vi "CAN CONF.vi"() -> ()   [LabVIEW 2018]
uses:
  Controls/CLUSTER.ctl
  Controls/FEV_DBC CLUSTER.ctl
  Controls/DBC CLUSTER.ctl
  <resource>/objmgr/xnet.rc
panel:
  out "File paths.Model File path":path
  out "appended path":path
  in  "DBC FUNCTIONS":T1[](array[typedef])
  out "Headline":string
  in  "ADD":bool
  in  "Save Button":bool
  in  "ALL DBC FUNCTIONS":T3[](array[typedef])
  in  "DBC File Selection":refnum<k21>="CAN DATA"
  out "Frames":refnum<k21>[](array[refnum])
  in  "MODEL SELECTION":string(combo)
  # "FUNCTIONS"
  # "FUNCTIONS"
  # "READ"
  # "WRITE"
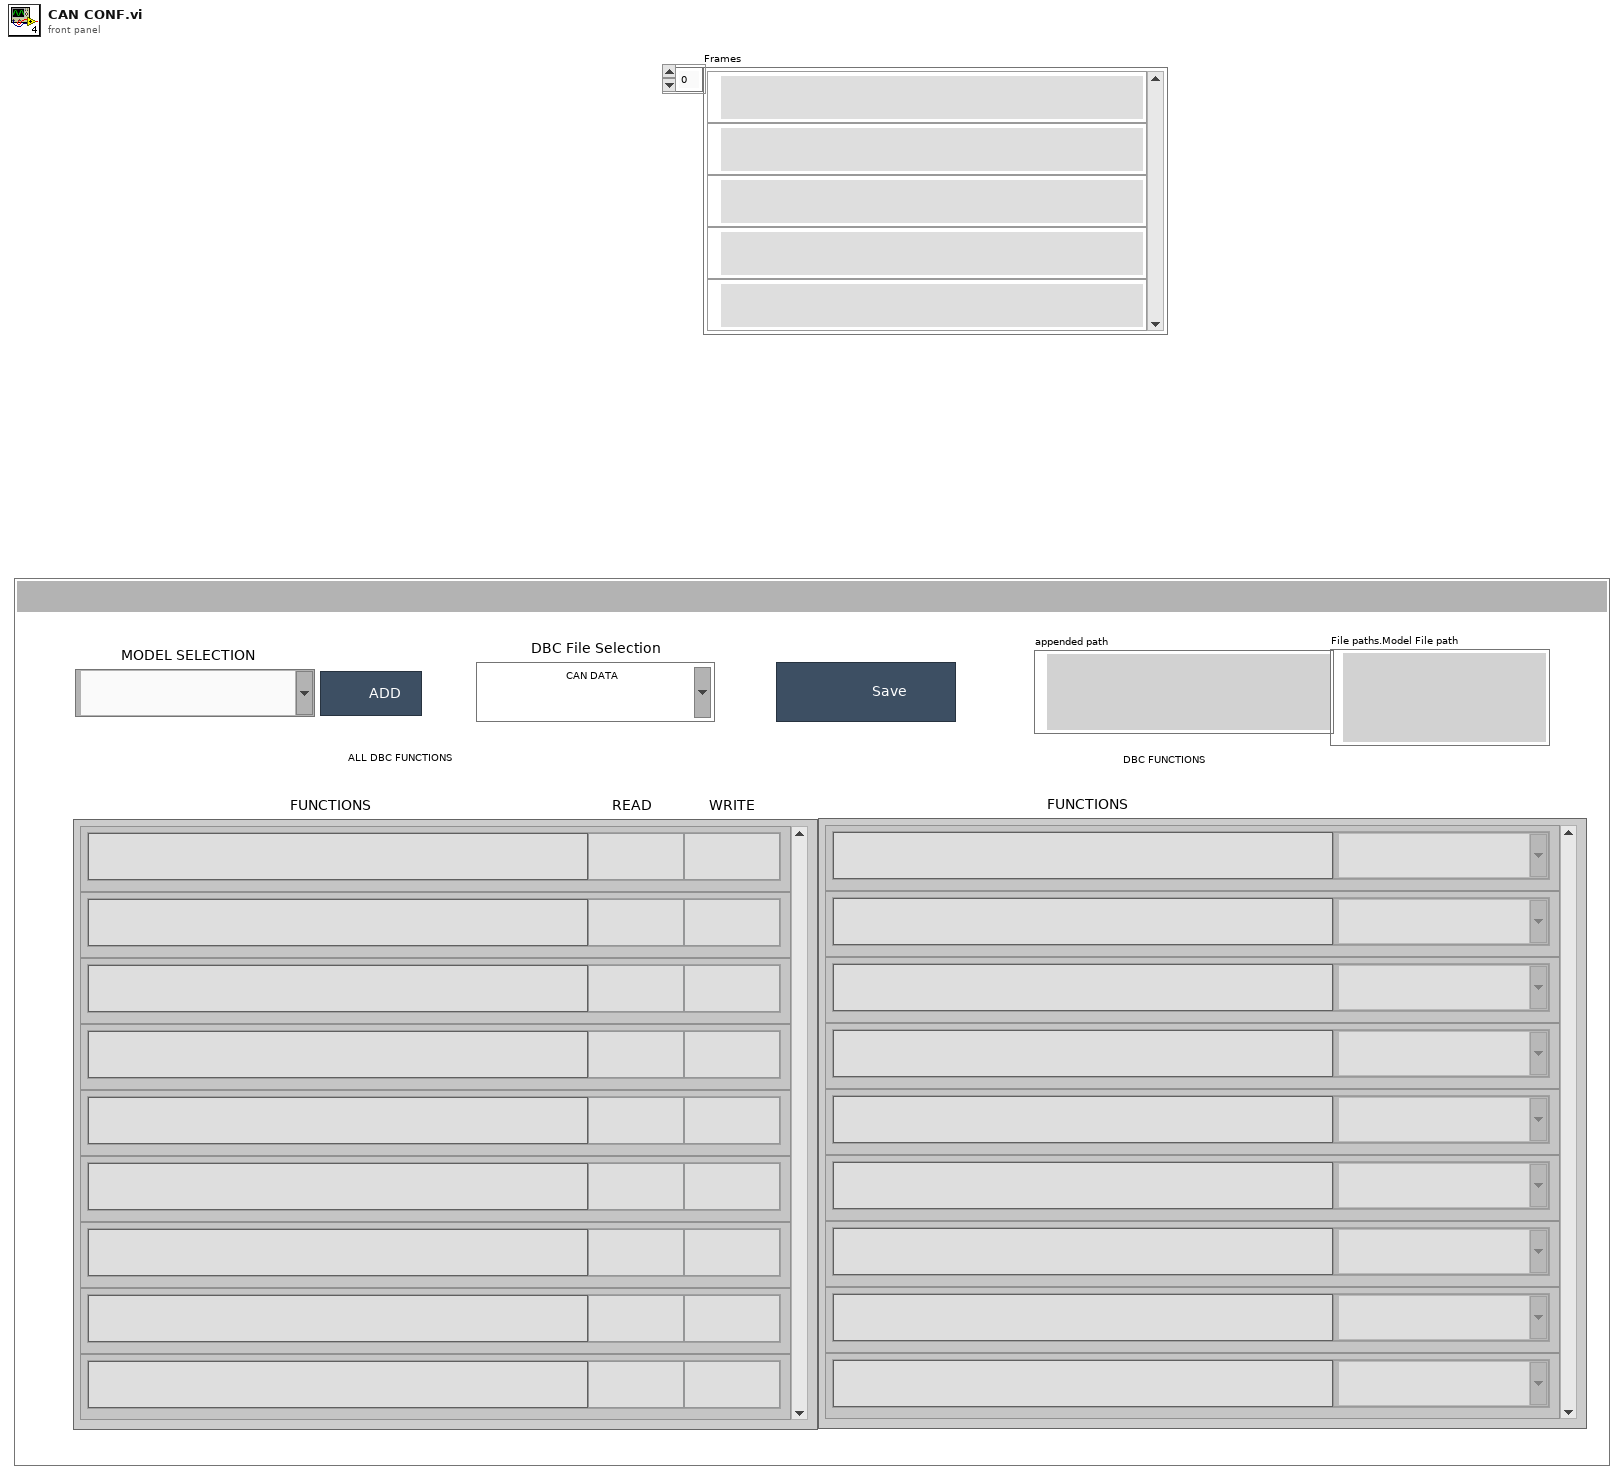
[diagram p1: front panel]
types:
  T1 = typedef "FEV_DBC CLUSTER.ctl" = cluster{"FUNCTION":T2, "DYNO FUNCTION":string}
  T2 = typedef "DBC CLUSTER.ctl" = string
  T3 = typedef "CLUSTER.ctl" = cluster{"FUNCTION":string, "READ":bool, "WRITE":bool}
  T4 = enum32{"Invalid", "Standard", "Closed", "Hidden", "Minimized", "Maximized"}
  T5 = enum32{"invalid app kind", "Development System", "Run Time System", "Student Edition", "Embedded LabVIEW", "Evaluation", "Custom"}
  T6 = cluster{"Core":cluster{"Current VI Reference":refnum<vi>, "Close Panel on Exit?":bool}, "Your Boolean data":bool, "Your string data":string, "ALL DBC FUNCTIONS":T3[], "File paths":cluster{"Base file path":path, "Model File path":path}, "DBC FUNCTIONS":T1[]}
  T7 = cluster{"Base file path":path, "Model File path":path}
  T8 = cluster{"Current VI Reference":refnum<vi>, "Close Panel on Exit?":bool}
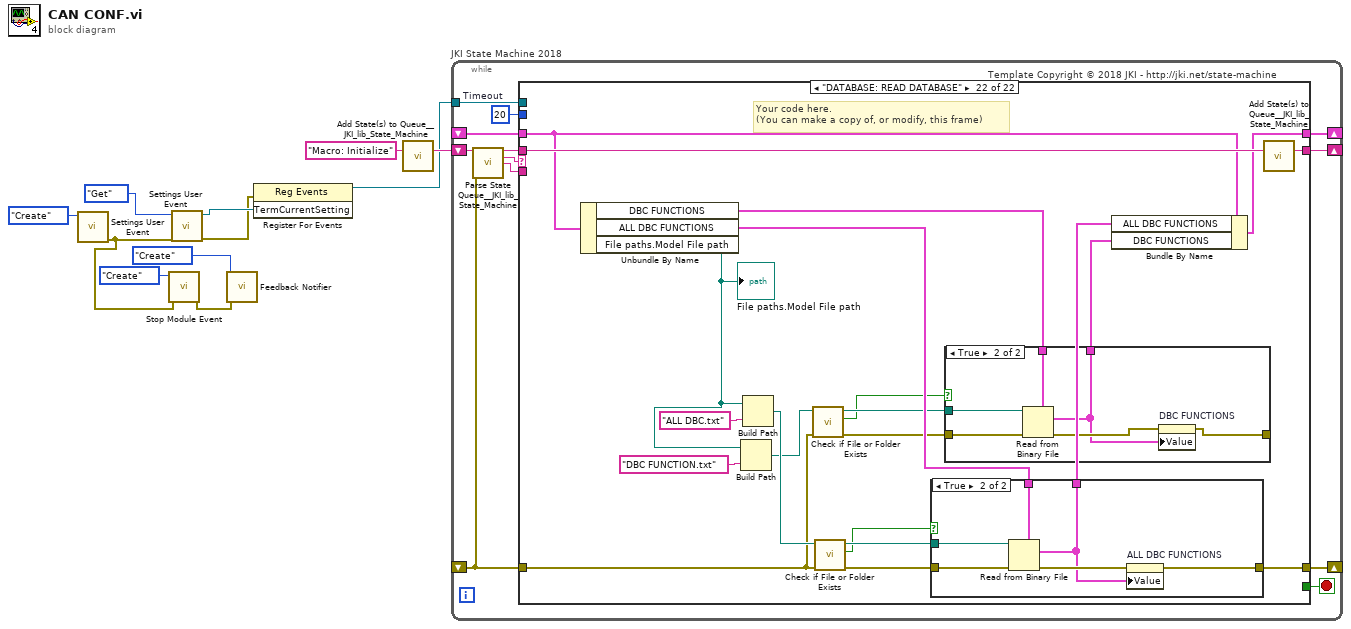
[diagram p0: block diagram]
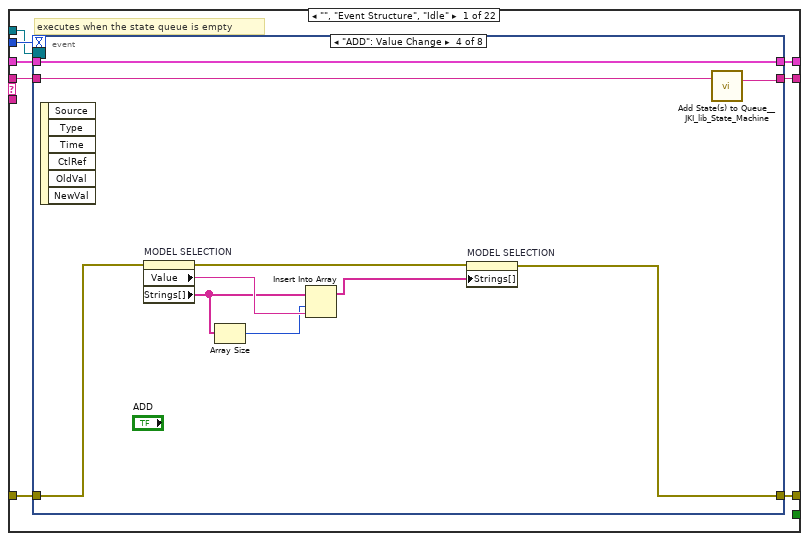
[diagram p2: hidden frame]
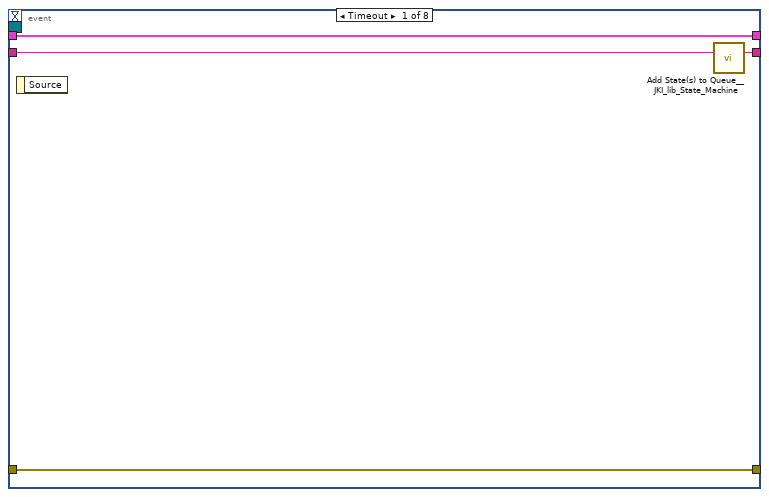
[diagram p3: hidden frame]
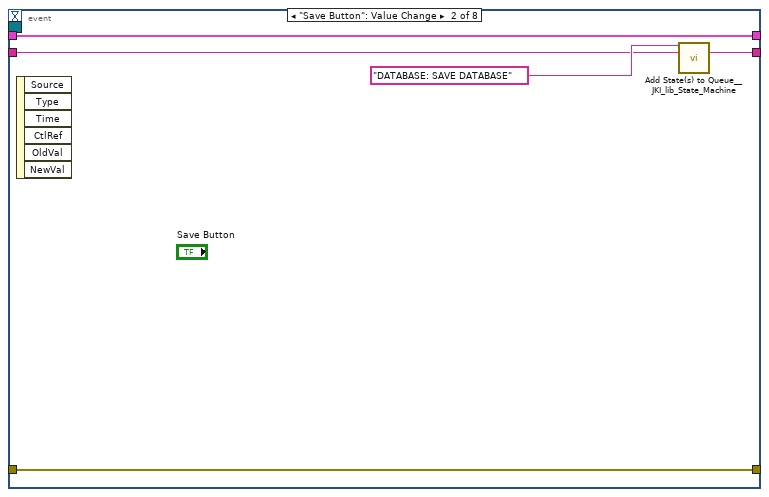
[diagram p4: hidden frame]
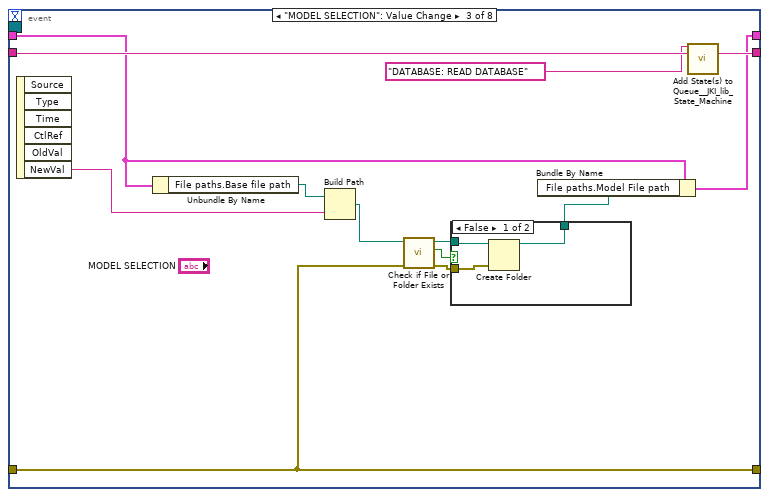
[diagram p5: hidden frame]
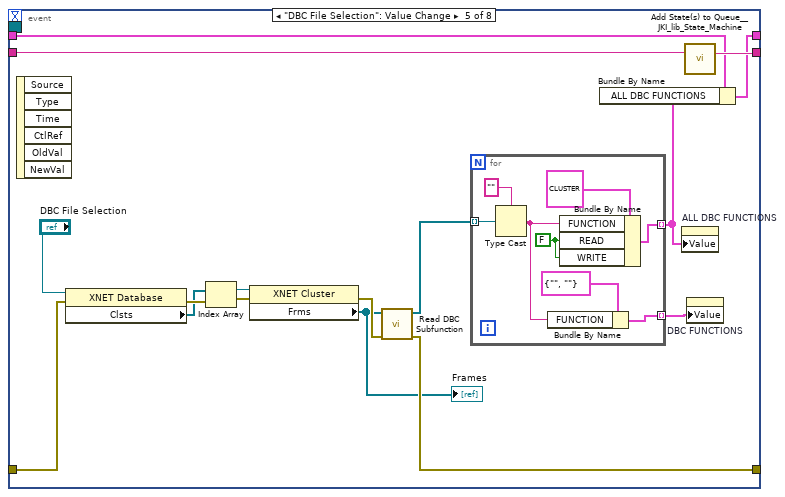
[diagram p7: hidden frame]
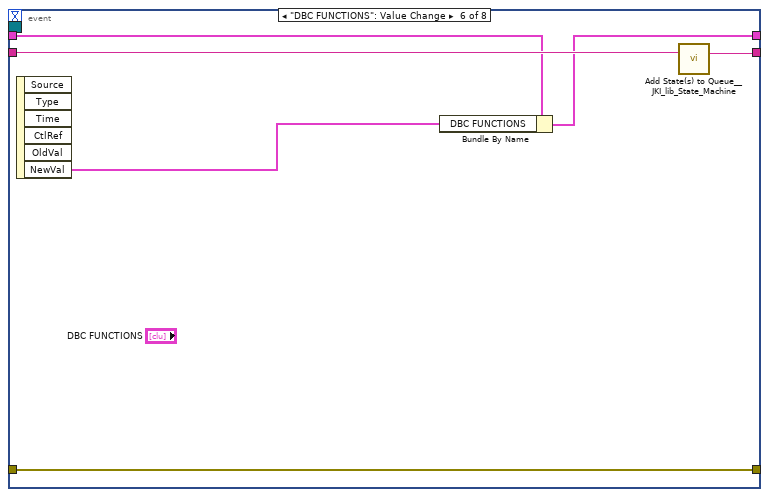
[diagram p8: hidden frame]
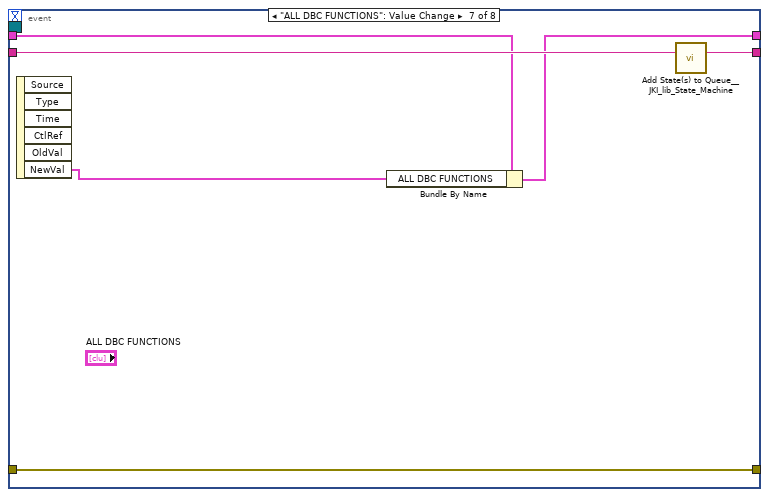
[diagram p9: hidden frame]
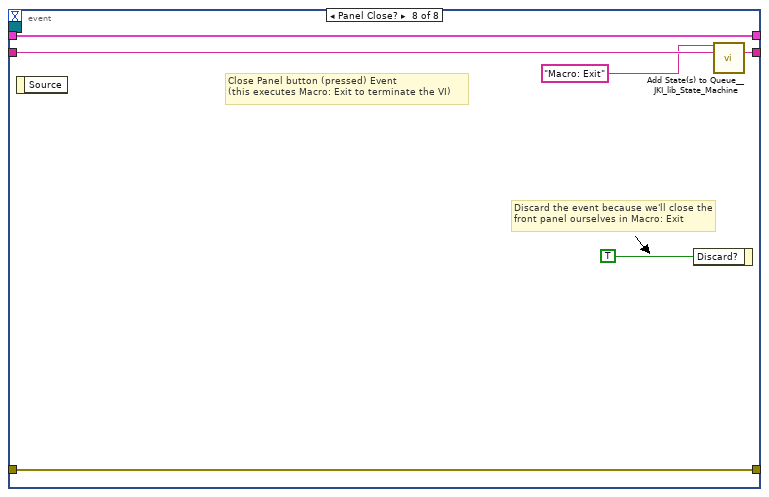
[diagram p10: hidden frame]
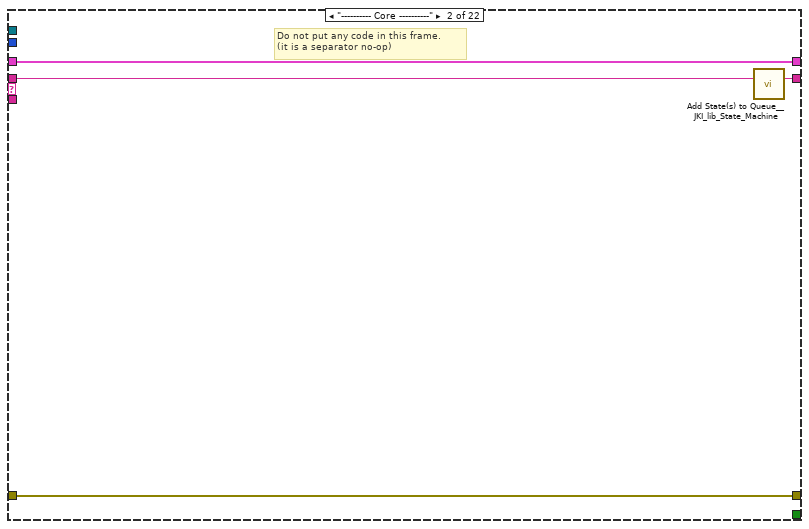
[diagram p11: hidden frame]
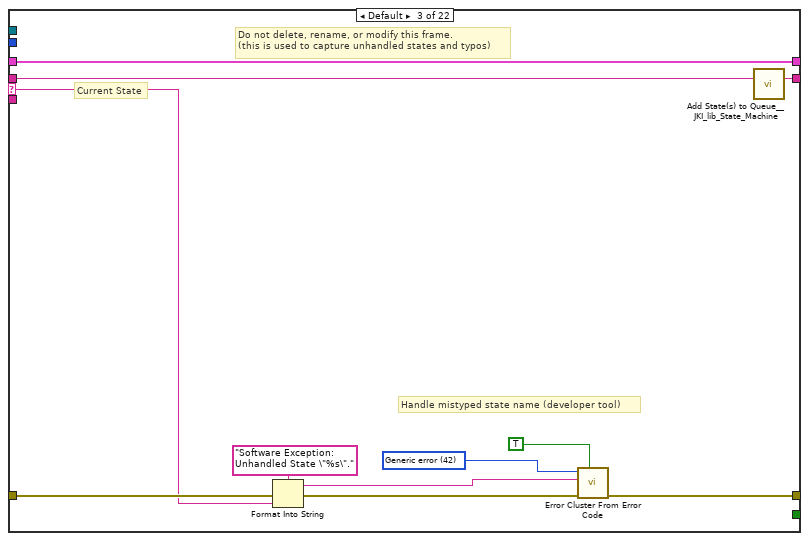
[diagram p12: hidden frame]
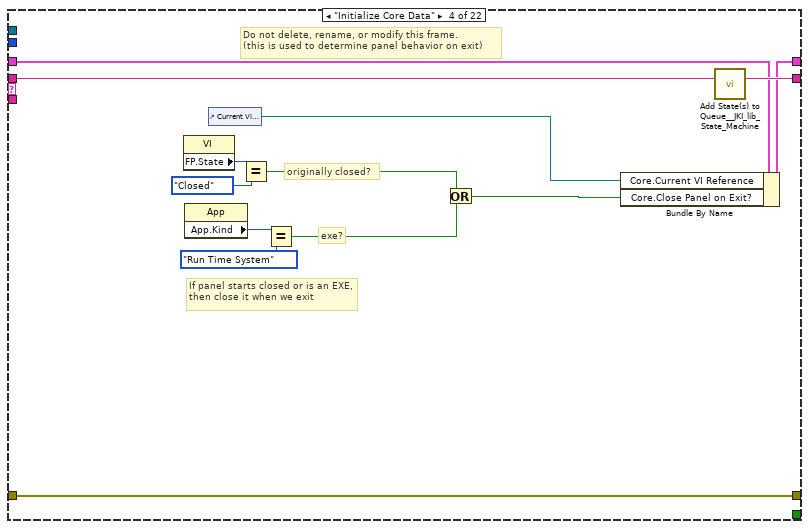
[diagram p13: hidden frame]
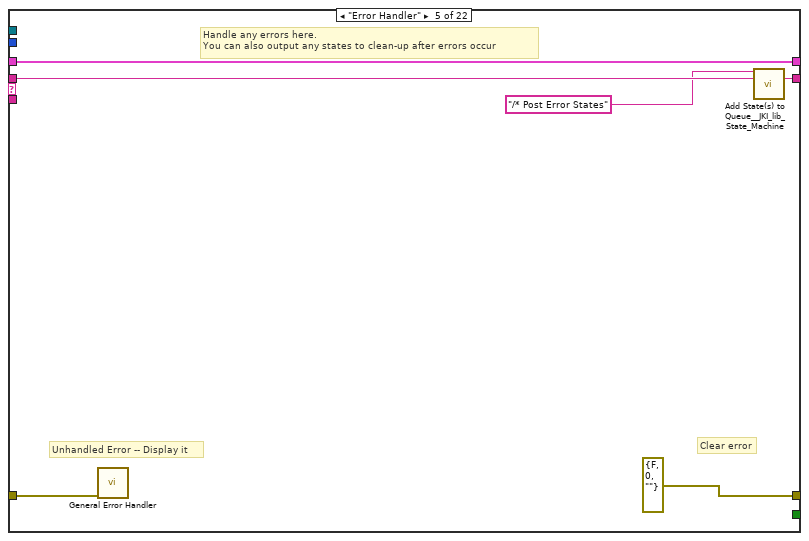
[diagram p14: hidden frame]
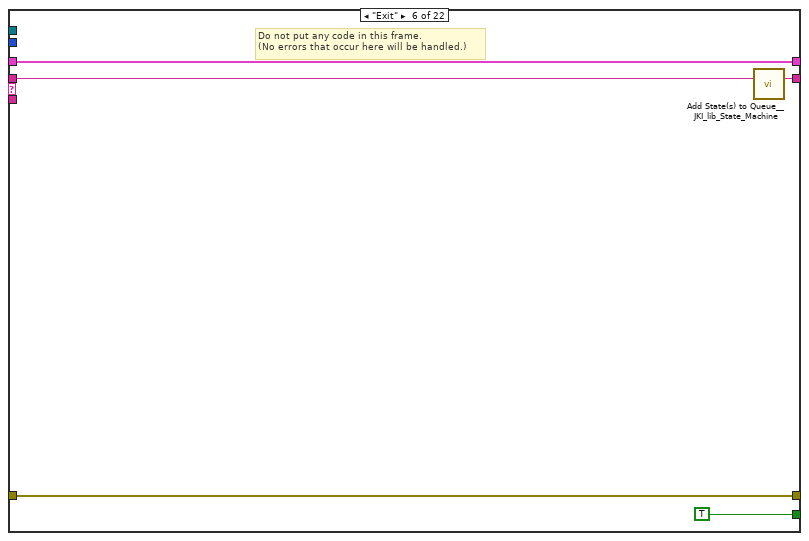
[diagram p15: hidden frame]
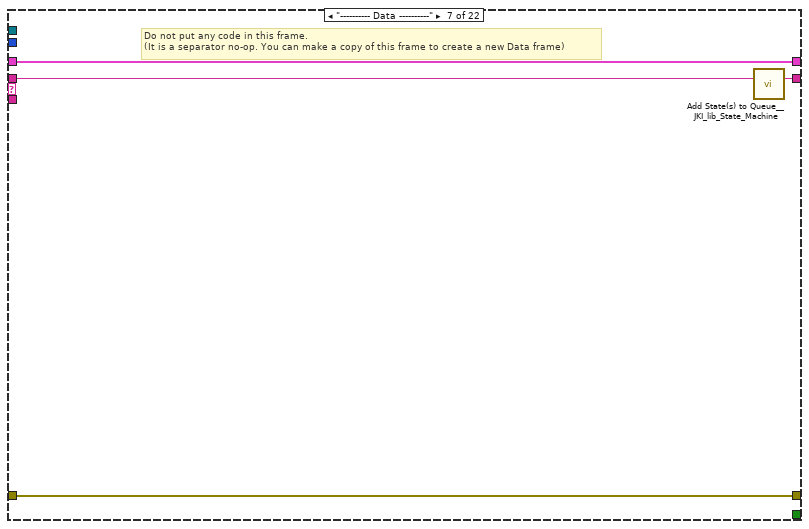
[diagram p16: hidden frame]
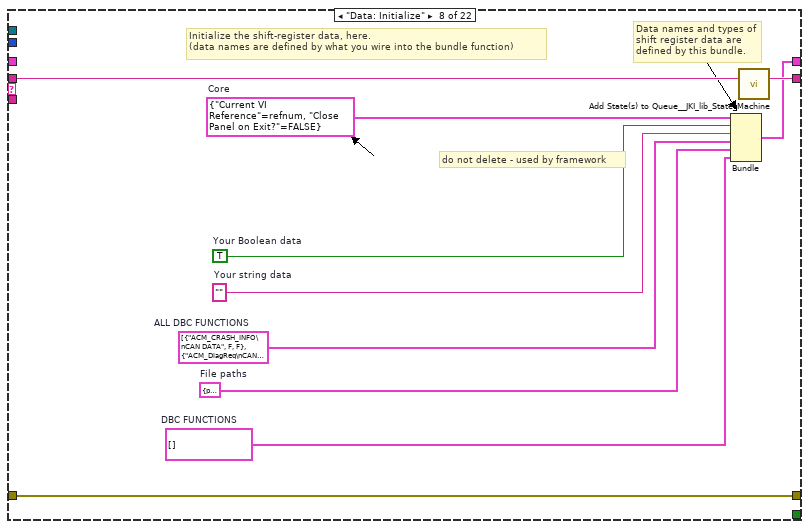
[diagram p17: hidden frame]
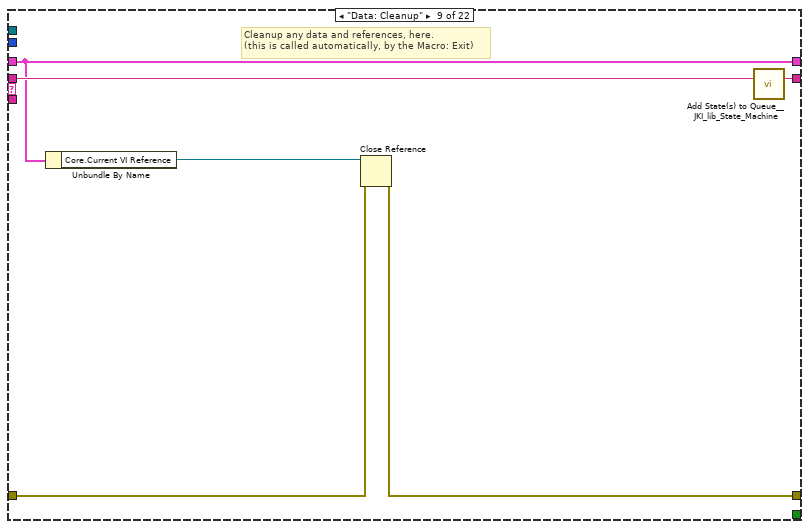
[diagram p18: hidden frame]
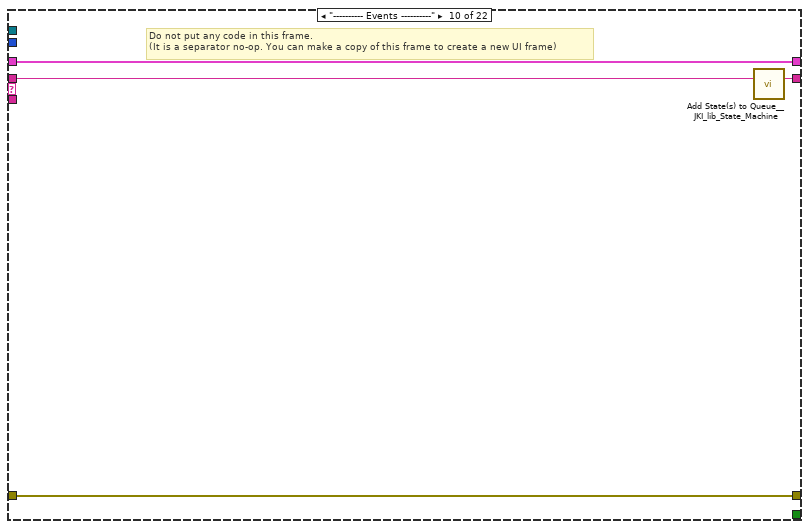
[diagram p19: hidden frame]
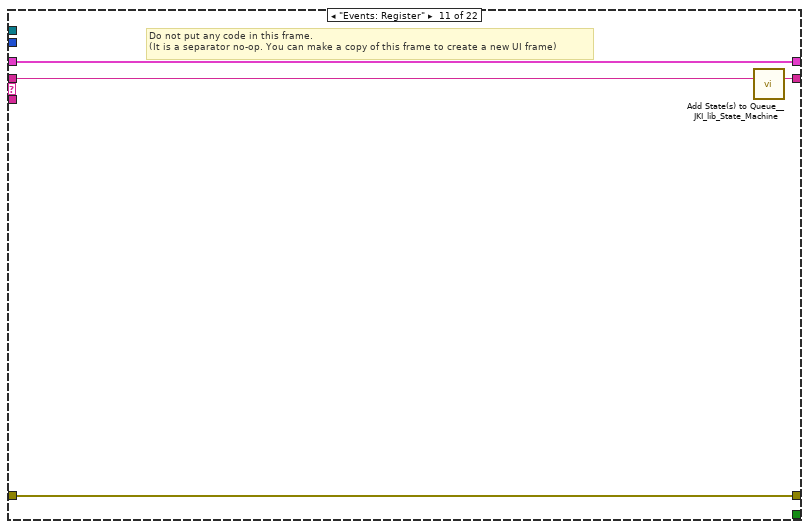
[diagram p20: hidden frame]
diagram:
  n1 = call "Settings User Event.vi"("Action"=enum16{"Create", "Get", "Destroy"}."Create") -> ("error out"=w4:errorcluster)  [unwired: 9 in, 1 out]
  n2 = call "Stop Module Event.vi"("error in (no error)"=w4, "Action"=enum16{"Create", "Get", "Destroy"}."Create") -> ("error out"=w3:errorcluster)  [unwired: 8 in, 1 out]
  n3 = call "Settings User Event.vi"("error in (no error)"=w4, "Action"=enum16{"Create", "Get", "Destroy"}."Get") -> ("error out"=w6:errorcluster, "TermCurrentSetting"=w7:refnum<user-event>)  [unwired: 8 in]
  n4 = call "Feedback Notifier.vi"("error in (no error)"=w3, "Action"=enum16{"Create", "Get", "Destroy"}."Create") -> ()  [unwired: 8 in, 2 out]
  n5 = register-events(error in=w6, w7) -> (reference out=w1:refnum<event-registration>)  [unwired: 1 in, 1 out]
  n6 = call <vilib>:"Add State(s) to Queue__JKI_lib_State_Machine.vi"("State(s) in (\"\")"="Macro: Initialize") -> ("States Out"=w11:string)  [unwired: 14 in]
  n7 = while "JKI State Machine 2018" {
    shift-right: [w16] -> _
    shift-left: _ -> [w15]
    shift-right: [w19] -> _
    shift-left: _ -> [w13]
    shift-right: [w18] -> _
    shift-left: w11 -> [w20]
    tunnel: w1 -> [w12]
    stop <- w17 stop-if-true
    w14 = 20  # Timeout
    # "Template Copyright © 2018 JKI - http://jki.net/state-machine"
    n8 = call <vilib>:"Parse State Queue__JKI_lib_State_Machine.vi"("State Queue"=w20, "Error In (no error)"=w13) -> ("Remaining States"=w22:string, "Current State"=w23:string, "Arguments"=w21:string)  [unwired: 11 in]
    n9 = case shown="\"DATABASE: READ DATABASE\"" w23 {
      selector: w23 -> [_ _ w113 _ _ _ _ _ _ _ _ _ _ _ _ _ _ _ _ _ _ _]
      tunnel: w22 -> [w31 w112 w117 w136 w142 w147 w151 w161 w167 w171 w175 w181 w185 w198 w204 w215 w284 w289 w299 w303 w317 w340]
      tunnel: w21 -> [_ _ _ _ _ _ _ _ _ _ _ _ _ _ w199 w209 _ _ _ _ _ _]
      tunnel: w15 -> [w29 w109 w115 w129 w139 w145 w148 _ w162 w168 w173 w179 w182 w192 w202 w211 w281 w286 w296 w300 w315 w336]
      tunnel: [w28 w110 w119 w133 errorcluster {"status"=FALSE, "code"=0, "source"=""} ("error out") w144 w149 w158 w163 w169 w172 w176 w183 w193 w200 w212 w282 w287 w297 w301 w306 w334] -> w19
      tunnel: w13 -> [w27 w110 w118 w133 w138 w144 w149 w158 w164 w169 w172 w177 w183 w190 w201 w213 w282 w287 w297 w301 w314 w325]
      tunnel: [w30 w111 w116 w135 w141 w146 w150 w160 w166 w170 w174 w180 w184 w197 w203 w214 w283 w288 w298 w302 w316 w339] -> w18
      tunnel: [_ _ _ _ _ TRUE _ _ _ _ _ _ _ _ _ _ _ _ _ _ _ _] -> w17
      tunnel: [w26 w109 w115 w134 w139 w145 w148 w159 w162 w168 w173 w179 w182 w191 w202 w211 w281 w286 w296 w300 w315 w335] -> w16
      tunnel: w14 -> [w25 _ _ _ _ _ _ _ _ _ _ _ _ _ _ _ _ _ _ _ _ _]
      tunnel: w12 -> [w24 _ _ _ _ _ _ _ _ _ _ w178 _ _ _ _ _ _ _ _ _ _]
      frame "", "Event Structure", "Idle" {
        # "executes when the state queue is empty"
        n10 = event shown="[3] \"ADD\": Value Change" {
          selector: w24 -> [_ _ _ _ _ _ _ _]
          dyn-events: _ -> [_ _ _ _ _ _ _ _]
          timeout: w25 -> [_ _ _ _ _ _ _ _]
          tunnel: w31 -> [w35 w37 w52 w58 w76 w94 w100 w108]
          tunnel: [w34 w38 w53 w59 w77 w95 w101 w107] -> w30
          tunnel: w29 -> [w32 w39 w48 w60 w75 w93 w99 w105]
          tunnel: [w33 w36 w45 w61 w70 w96 w102 w106] -> w28
          tunnel: w27 -> [w33 w36 w45 w67 w78 w96 w102 w106]
          tunnel: [w32 w39 w47 w60 w74 w91 w97 w105] -> w26
          event Timeout {
            n11 = event-data() -> ()  [unwired: 1 in, 1 out]
            n12 = call <vilib>:"Add State(s) to Queue__JKI_lib_State_Machine.vi"("State(s) in (\"\")"=w35) -> ("States Out"=w34:string)  [unwired: 14 in]
          }
          event "Save Button": Value Change {
            n13 = event-data() -> ()  [unwired: 1 in, 6 out]
            n14 = call <vilib>:"Add State(s) to Queue__JKI_lib_State_Machine.vi"("State(s) in Front (\"\")"="DATABASE: SAVE DATABASE", "State(s) in (\"\")"=w37) -> ("States Out"=w38:string)  [unwired: 13 in]
          }
          event "MODEL SELECTION": Value Change {
            n15 = event-data() -> ("NewVal"=w49:string)  [unwired: 1 in, 5 out]
            n16 = Unbundle By Name(w48) -> ("File paths.Base file path"=w50:path)
            n17 = Build Path(base path=w50, name or relative path=w49) -> (appended path=w46:path)
            n18 = call <vilib>:"Check if File or Folder Exists.vi"("error in (no error)"=w45, "path"=w46) -> ("error out"=w43:errorcluster, "file or folder exists?"=w42:bool, "dup path"=w44:path)  [unwired: 7 in]
            n19 = case shown="False" w42 {
              tunnel: w44 -> [w55 w57]
              tunnel: w43 -> [w56 _]
              tunnel: [w54 w57] -> w41
              frame False {
                n20 = Create Folder(path (use dialog)=w55, error in=w56) -> (created path=w54:path)  [unwired: 1 in, 2 out]
              }
              frame True {
              }
            }
            n21 = Bundle By Name(cluster=w48, "File paths.Model File path"=w41) -> (w47:T6)
            n22 = call <vilib>:"Add State(s) to Queue__JKI_lib_State_Machine.vi"("State(s) in Front (\"\")"="DATABASE: READ DATABASE", "State(s) in (\"\")"=w52) -> ("States Out"=w53:string)  [unwired: 13 in]
          }
          event "ADD": Value Change {
            n23 = event-data() -> ()  [unwired: 1 in, 6 out]
            n24 = property on="MODEL SELECTION" class="CmbBox"(error in=w67) -> (error out=w66:errorcluster, "Value"=w65:string, "Strings[]"=w64:string[])  [unwired: 1 in, 1 out]
            n25 = Array Size(array=w64) -> (size(s)=w63:i32)
            n26 = Insert Into Array(array=w64, index=w63, new element=w65) -> (w62:string[])
            n27 = property on="MODEL SELECTION" class="CmbBox"(error in=w66, "Strings[]"=w62) -> (error out=w61:errorcluster)  [unwired: 1 in, 1 out]
            n28 = call <vilib>:"Add State(s) to Queue__JKI_lib_State_Machine.vi"("State(s) in (\"\")"=w58) -> ("States Out"=w59:string)  [unwired: 14 in]
          }
          event "DBC File Selection": Value Change {
            n29 = event-data() -> ()  [unwired: 1 in, 6 out]
            n30 = property class="XNET Database"(reference="DBC File Selection", error in=w78) -> (error out=w81:errorcluster, "Clsts"=w80:refnum<k21>[])  [unwired: 1 out]
            n31 = Index Array(array=w80) -> (element=w82:refnum<k21>)  [unwired: 1 in]
            n32 = property class="XNET Cluster"(reference=w82, error in=w81) -> (error out=w71:errorcluster, "Frms"=w68:refnum<k21>[])  [unwired: 1 out]
            "Frames" <- w68
            n33 = call "Read DBC Subfunction.vi"("error In"=w71, "Frames"=w68) -> ("error out"=w70:errorcluster, "Sigs"=w69:refnum<k21>[])  [unwired: 8 in]
            n34 = for {
              tunnel: [w89] -> w73 mode=indexing
              tunnel: w69 -> [w86] mode=indexing
              tunnel: [w83] -> w72 mode=indexing
              w87 = FALSE ("READ")
              n35 = Type Cast(type="" ("FUNCTION"), x=w86) -> (*(type *) &x=w84:string)
              n36 = Bundle By Name(cluster=T1 {"FUNCTION"="", "DYNO FUNCTION"=""} ("FUNCTIONS"), "FUNCTION"=w84) -> (w83:T1)
              n37 = Bundle By Name(cluster=T3 {"FUNCTION"="ACM_CRASH_INFO\nCAN DATA", "READ"=TRUE, "WRITE"=TRUE} ("FUNCTIONS"), "FUNCTION"=w84, "READ"=w87, "WRITE"=w87) -> (w89:T3)
            }
            n38 = Bundle By Name(cluster=w75, "ALL DBC FUNCTIONS"=w73) -> (w74:T6)
            n39 = property on="ALL DBC FUNCTIONS" class="Arr (strict)"("Value"=w73) -> ()  [unwired: 2 in, 2 out]
            n40 = call <vilib>:"Add State(s) to Queue__JKI_lib_State_Machine.vi"("State(s) in (\"\")"=w76) -> ("States Out"=w77:string)  [unwired: 14 in]
            n41 = property on="DBC FUNCTIONS" class="Arr (strict)"("Value"=w72) -> ()  [unwired: 2 in, 2 out]
          }
          event "DBC FUNCTIONS": Value Change {
            n42 = event-data() -> ("NewVal"=w92:T1[])  [unwired: 1 in, 5 out]
            n43 = Bundle By Name(cluster=w93, "DBC FUNCTIONS"=w92) -> (w91:T6)
            n44 = call <vilib>:"Add State(s) to Queue__JKI_lib_State_Machine.vi"("State(s) in (\"\")"=w94) -> ("States Out"=w95:string)  [unwired: 14 in]
          }
          event "ALL DBC FUNCTIONS": Value Change {
            n45 = event-data() -> ("NewVal"=w98:T3[])  [unwired: 1 in, 5 out]
            n46 = Bundle By Name(cluster=w99, "ALL DBC FUNCTIONS"=w98) -> (w97:T6)
            n47 = call <vilib>:"Add State(s) to Queue__JKI_lib_State_Machine.vi"("State(s) in (\"\")"=w100) -> ("States Out"=w101:string)  [unwired: 14 in]
          }
          event Panel Close? {
            # "Discard the event because we'll close the front panel ourselves in Macro: Exit"
            # "Close Panel button (pressed) Event\n(this executes Macro: Exit to terminate the VI)"
            n48 = event-data() -> ()  [unwired: 1 in, 1 out]
            n49 = event-data("Discard?"=TRUE) -> ()  [unwired: 1 in, 1 out]
            n50 = call <vilib>:"Add State(s) to Queue__JKI_lib_State_Machine.vi"("State(s) in Front (\"\")"="Macro: Exit", "State(s) in (\"\")"=w108) -> ("States Out"=w107:string)  [unwired: 13 in]
          }
        }
      }
      frame "---------- Core ----------" {
        # "Do not put any code in this frame.\n(it is a separator no-op)"
        n51 = call <vilib>:"Add State(s) to Queue__JKI_lib_State_Machine.vi"("State(s) in (\"\")"=w112) -> ("States Out"=w111:string)  [unwired: 14 in]
      }
      frame Default {
        w122 = 42 items=["No error", "Argument error", "Memory is full", "Out of zone", "End of file", "File already open", "Generic file I/O error", "File not found", "File permission error", "Disk is full", "Duplicate path", "Too many files open", "System feature not enabled", "Resource file not found", "Cannot add resource", "Resource not found", "Image not found", "Image memory error", "Pen does not exist", "Config type invalid", "Config token not found", "Config parse error", "Config memory error", "Bad external code format", "Bad external code offset", "External code not present", "Null window", "Destroy window error", "Null menu", "Print aborted", "Bad print record", "Print driver error", "Windows error during printing", "Memory error during printing", "Print dialog error", "Generic print error", "Invalid device refnum", "Device not found", "Device parameter error", "Device unit error", "Cannot open device", "Device call aborted", "Generic error", "Cancelled by user", "Object ID too low", "Object ID too high", "Object not in heap", "Unknown heap", "Unknown object (invalid DefProc)", "Unknown object (DefProc not in table)", "Message out of range", "Invalid (null) method", "Unknown message", "Manager call not supported", "Bad address", "Network operation in progress", "Network operation timed out", "Connection is busy", "Network attribute not supported", "Network error", "Address in use", "System out of memory", "Connection aborted", "Connection refused", "Not connected", "Already connected", "Connection closed", "Initialization error (interapplication manager)", "Bad occurrence", "Wait on unbound occurrence handler", "Occurrence queue overflow", "Datalog type conflict", "Unused", "Unrecognized type (interapplication manager)", "Memory corrupt", "Failed to make temporary DLL", "Old CIN version", "Drag socket not found", "Failed to load drop-object", "Failed to register OLE object", "Failed to release OLE object", "Format specifier type mismatch", "Unknown format specifier", "Too few format specifiers", "Too many format specifiers", "Scan failed", "Newer CIN version", "Error converting to variant", "Runtime menu error", "Password tampered", "Variant attribute not found", "Incompatible variant data type", "Event data is not available", "Event Store is not present", "Occurrence is not found", "Event Queue is not created", "Event info is not available", "Refnum passed is NULL", "Error retrieving Class GUID", "Error retrieving CoClass GUID", "Error retrieving TypeLib GUID.", "Bad built application magic bytes.", "Specific driver is different from the specific driver associated with the Logical Name.", "There is no session opened to the class driver.", "Max Error", "MAX - Error with config objects", "MAX - Error loading configuration", "MAX - Group not supported"]
        # "Current State"
        # "Do not delete, rename, or modify this frame.\n(this is used to capture unhandled states and typos)"
        # "Handle mistyped state name (developer tool)"
        n52 = Format Into String(format string="Software Exception: Unhandled State \"%s\"." ("message"), error in=w118, w113) -> (resulting string=w121:string, error out=w120:errorcluster)  [unwired: 1 in]
        n53 = call <vilib>:"Error Cluster From Error Code.vi"("show call chain? (False)"=TRUE, "error in (no error)"=w120, "error message (\"\")"=w121, "error code (0)"=w122) -> ("error out"=w119:errorcluster)  [unwired: 5 in]
        n54 = call <vilib>:"Add State(s) to Queue__JKI_lib_State_Machine.vi"("State(s) in (\"\")"=w117) -> ("States Out"=w116:string)  [unwired: 14 in]
      }
      frame "Initialize Core Data" {
        # "Do not delete, rename, or modify this frame.\n(this is used to determine panel behavior on exit)"
        # "originally closed?"
        # "exe?"
        # "If panel starts closed or is an EXE, then close it when we exit"
        n55 = property class="VI"() -> ("FP.State"=w126:T4)  [unwired: 2 in, 2 out]
        n56 = property class="App"() -> ("App.Kind"=w132:T5)  [unwired: 2 in, 2 out]
        n57 = control-ref of="Current VI Reference"() -> (w127:refnum<vi>)
        n58 = Equal?(x=w126, y=T4."Closed" ("Front Panel Window:State")) -> (x = y?=w124:bool)
        n59 = Equal?(x=w132, y=T5."Run Time System" ("Application:Kind")) -> (x = y?=w130:bool)
        n60 = Or(x=w124, y=w130) -> (x .or. y?=w128:bool)
        n61 = Bundle By Name(cluster=w129, "Core.Current VI Reference"=w127, "Core.Close Panel on Exit?"=w128) -> (w134:T6)
        n62 = call <vilib>:"Add State(s) to Queue__JKI_lib_State_Machine.vi"("State(s) in (\"\")"=w136) -> ("States Out"=w135:string)  [unwired: 14 in]
      }
      frame "Error Handler" {
        # "Unhandled Error -- Display it"
        # "Handle any errors here.\nYou can also output any states to clean-up after errors occur"
        # "Clear error"
        n63 = call <vilib>:"General Error Handler.vi"("error in (no error)"=w138) -> ()  [unwired: 10 in, 5 out]
        n64 = call <vilib>:"Add State(s) to Queue__JKI_lib_State_Machine.vi"("State(s) in Front (\"\")"="/* Post Error States", "State(s) in (\"\")"=w142) -> ("States Out"=w141:string)  [unwired: 13 in]
      }
      frame "Exit" {
        # "Do not put any code in this frame.\n(No errors that occur here will be handled.)"
        n65 = call <vilib>:"Add State(s) to Queue__JKI_lib_State_Machine.vi"("State(s) in (\"\")"=w147) -> ("States Out"=w146:string)  [unwired: 14 in]
      }
      frame "---------- Data ----------" {
        # "Do not put any code in this frame.\n(It is a separator no-op. You can make a copy of this frame to create a new Data frame)"
        n66 = call <vilib>:"Add State(s) to Queue__JKI_lib_State_Machine.vi"("State(s) in (\"\")"=w151) -> ("States Out"=w150:string)  [unwired: 14 in]
      }
      frame "Data: Initialize" {
        w152 = T1[] []  # DBC FUNCTIONS
        w153 = T7 {"Base file path"=path "", "Model File path"=path ""}  # File paths
        w154 = T3[] [{"FUNCTION"="ACM_CRASH_INFO\nCAN DATA", "READ"=FALSE, "WRITE"=FALSE}, {"FUNCTION"="ACM_DiagReq\nCAN DATA", "READ"=FALSE, "WRITE"=FALSE}, {"FUNCTION"="ACM_DiagResp\nCAN DATA", "READ"=FALSE, "WRITE"=FALSE}, {"FUNCTION"="ACM_OCCUPANT_STATUS\nCAN DATA", "READ"=FALSE, "WRITE"=FALSE}, {"FUNCTION"="ACM_WarnMsg\nCAN DATA", "READ"=FALSE, "WRITE"=FALSE}, {"FUNCTION"="ADAS_AEB\nCAN DATA", "READ"=FALSE, "WRITE"=FALSE}, {"FUNCTION"="ADAS_AHB_DOW\nCAN DATA", "READ"=FALSE, "WRITE"=FALSE}, {"FUNCTION"="ADAS_APA_SLOT1INFO1\nCAN DATA", "READ"=FALSE, "WRITE"=FALSE}, {"FUNCTION"="ADAS_APA_SLOT1INFO2\nCAN DATA", "READ"=FALSE, "WRITE"=FALSE}, {"FUNCTION"="ADAS_APA_SLOT1INFO3\nCAN DATA", "READ"=FALSE, "WRITE"=FALSE}, {"FUNCTION"="ADAS_APA_SLOT2INFO1\nCAN DATA", "READ"=FALSE, "WRITE"=FALSE}, {"FUNCTION"="ADAS_APA_SLOT2INFO2\nCAN DATA", "READ"=FALSE, "WRITE"=FALSE}, {"FUNCTION"="ADAS_APA_SLOT2INFO3\nCAN DATA", "READ"=FALSE, "WRITE"=FALSE}, {"FUNCTION"="ADAS_APA_SLOT3INFO1\nCAN DATA", "READ"=FALSE, "WRITE"=FALSE}, {"FUNCTION"="ADAS_APA_SLOT3INFO2\nCAN DATA", "READ"=FALSE, "WRITE"=FALSE}, {"FUNCTION"="ADAS_APA_SLOT3INFO3\nCAN DATA", "READ"=FALSE, "WRITE"=FALSE}, {"FUNCTION"="ADAS_APA_SLOT4INFO1\nCAN DATA", "READ"=FALSE, "WRITE"=FALSE}, {"FUNCTION"="ADAS_APA_SLOT4INFO2\nCAN DATA", "READ"=FALSE, "WRITE"=FALSE}, {"FUNCTION"="ADAS_APA_SLOT4INFO3\nCAN DATA", "READ"=FALSE, "WRITE"=FALSE}, {"FUNCTION"="ADAS_APA_SLOT5INFO1\nCAN DATA", "READ"=FALSE, "WRITE"=FALSE}, {"FUNCTION"="ADAS_APA_SLOT5INFO2\nCAN DATA", "READ"=FALSE, "WRITE"=FALSE}, {"FUNCTION"="ADAS_APA_SLOT5INFO3\nCAN DATA", "READ"=FALSE, "WRITE"=FALSE}, {"FUNCTION"="ADAS_APA_SLOT6INFO1\nCAN DATA", "READ"=FALSE, "WRITE"=FALSE}, {"FUNCTION"="ADAS_APA_SLOT6INFO2\nCAN DATA", "READ"=FALSE, "WRITE"=FALSE}, {"FUNCTION"="ADAS_APA_SLOT6INFO3\nCAN DATA", "READ"=FALSE, "WRITE"=FALSE}, {"FUNCTION"="ADAS_AVM_Sts\nCAN DATA", "READ"=FALSE, "WRITE"=FALSE}, {"FUNCTION"="ADAS_BSD\nCAN DATA", "READ"=FALSE, "WRITE"=FALSE}, {"FUNCTION"="ADAS_CMP_ACC\nCAN DATA", "READ"=FALSE, "WRITE"=FALSE}, {"FUNCTION"="ADAS_CMP_CHECK\nCAN DATA", "READ"=FALSE, "WRITE"=FALSE}, {"FUNCTION"="ADAS_CMP_MHU\nCAN DATA", "READ"=FALSE, "WRITE"=FALSE}, {"FUNCTION"="ADAS_DMS_STATUS\nCAN DATA", "READ"=FALSE, "WRITE"=FALSE}, {"FUNCTION"="ADAS_DiagReq\nCAN DATA", "READ"=FALSE, "WRITE"=FALSE}, {"FUNCTION"="ADAS_DiagResp\nCAN DATA", "READ"=FALSE, "WRITE"=FALSE}, {"FUNCTION"="ADAS_ELK\nCAN DATA", "READ"=FALSE, "WRITE"=FALSE}, {"FUNCTION"="ADAS_FCW_RCTA\nCAN DATA", "READ"=FALSE, "WRITE"=FALSE}, {"FUNCTION"="ADAS_Immo_MHU\nCAN DATA", "READ"=FALSE, "WRITE"=FALSE}, {"FUNCTION"="ADAS_LDW_LKA\nCAN DATA", "READ"=FALSE, "WRITE"=FALSE}, {"FUNCTION"="ADAS_NM\nCAN DATA", "READ"=FALSE, "WRITE"=FALSE}, {"FUNCTION"="ADAS_PA\nCAN DATA", "READ"=FALSE, "WRITE"=FALSE}, {"FUNCTION"="ADAS_RP_Sts\nCAN DATA", "READ"=FALSE, "WRITE"=FALSE}, {"FUNCTION"="ADAS_Speed_Display\nCAN DATA", "READ"=FALSE, "WRITE"=FALSE}, {"FUNCTION"="ADAS_TSR_STATUS\nCAN DATA", "READ"=FALSE, "WRITE"=FALSE}, {"FUNCTION"="ADAS_WarnMsg\nCAN DATA", "READ"=FALSE, "WRITE"=FALSE}, {"FUNCTION"="AMP_DiagReq\nCAN DATA", "READ"=FALSE, "WRITE"=FALSE}, {"FUNCTION"="AMP_DiagResp\nCAN DATA", "READ"=FALSE, "WRITE"=FALSE}, {"FUNCTION"="AMP_MHUEQType\nCAN DATA", "READ"=FALSE, "WRITE"=FALSE}, {"FUNCTION"="AMP_MHU_Ann1_ModeSET\nCAN DATA", "READ"=FALSE, "WRITE"=FALSE}, {"FUNCTION"="AMP_MHU_Ann1_PromptsSET\nCAN DATA", "READ"=FALSE, "WRITE"=FALSE}, {"FUNCTION"="AMP_MHU_Ann2_SpeakerSET\nCAN DATA", "READ"=FALSE, "WRITE"=FALSE}, {"FUNCTION"="AMP_MHU_SET\nCAN DATA", "READ"=FALSE, "WRITE"=FALSE}, {"FUNCTION"="AMP_NM\nCAN DATA", "READ"=FALSE, "WRITE"=FALSE}, {"FUNCTION"="AMP_rDiagReq\nCAN DATA", "READ"=FALSE, "WRITE"=FALSE}, {"FUNCTION"="AMP_rDiagResp\nCAN DATA", "READ"=FALSE, "WRITE"=FALSE}, {"FUNCTION"="APA_FEEDBACK_MHU\nCAN DATA", "READ"=FALSE, "WRITE"=FALSE}, {"FUNCTION"="APA_SENSOR\nCAN DATA", "READ"=FALSE, "WRITE"=FALSE}, {"FUNCTION"="APM_DiagReq\nCAN DATA", "READ"=FALSE, "WRITE"=FALSE}, {"FUNCTION"="APM_DiagResp\nCAN DATA", "READ"=FALSE, "WRITE"=FALSE}, {"FUNCTION"="APM_WINDOW_POS\nCAN DATA", "READ"=FALSE, "WRITE"=FALSE}, {"FUNCTION"="APM_WarnMsg\nCAN DATA", "READ"=FALSE, "WRITE"=FALSE}, {"FUNCTION"="ASU_DiagReq\nCAN DATA", "READ"=FALSE, "WRITE"=FALSE}, {"FUNCTION"="ASU_DiagResp\nCAN DATA", "READ"=FALSE, "WRITE"=FALSE}, {"FUNCTION"="AVAS_DiagReq\nCAN DATA", "READ"=FALSE, "WRITE"=FALSE}, {"FUNCTION"="AVAS_DiagResp\nCAN DATA", "READ"=FALSE, "WRITE"=FALSE}, {"FUNCTION"="AVAS_STATUS\nCAN DATA", "READ"=FALSE, "WRITE"=FALSE}, {"FUNCTION"="BCM_ALM_warning\nCAN DATA", "READ"=FALSE, "WRITE"=FALSE}, {"FUNCTION"="BCM_BPM_DiagReq\nCAN DATA", "READ"=FALSE, "WRITE"=FALSE}, {"FUNCTION"="BCM_BPM_DiagResp\nCAN DATA", "READ"=FALSE, "WRITE"=FALSE}, {"FUNCTION"="BCM_CLAMP_STAT\nCAN DATA", "READ"=FALSE, "WRITE"=FALSE}, {"FUNCTION"="BCM_Comfort_Confirm_sts\nCAN DATA", "READ"=FALSE, "WRITE"=FALSE}, {"FUNCTION"="BCM_DiagReq\nCAN DATA", "READ"=FALSE, "WRITE"=FALSE}, {"FUNCTION"="BCM_DiagResp\nCAN DATA", "READ"=FALSE, "WRITE"=FALSE}, {"FUNCTION"="BCM_ENERGY_MANAGEMENT\nCAN DATA", "READ"=FALSE, "WRITE"=FALSE}, {"FUNCTION"="BCM_ENTRY_CONTROL\nCAN DATA", "READ"=FALSE, "WRITE"=FALSE}, {"FUNCTION"="BCM_FKS_STATUS\nCAN DATA", "READ"=FALSE, "WRITE"=FALSE}, {"FUNCTION"="BCM_LIGHT\nCAN DATA", "READ"=FALSE, "WRITE"=FALSE}, {"FUNCTION"="BCM_LOGICAL_CLAMP\nCAN DATA", "READ"=FALSE, "WRITE"=FALSE}, {"FUNCTION"="BCM_Mirror_Confirm_sts\nCAN DATA", "READ"=FALSE, "WRITE"=FALSE}, {"FUNCTION"="BCM_ODO\nCAN DATA", "READ"=FALSE, "WRITE"=FALSE}, {"FUNCTION"="BCM_RainLightSnr\nCAN DATA", "READ"=FALSE, "WRITE"=FALSE}, {"FUNCTION"="BCM_SCM_LIN_Info\nCAN DATA", "READ"=FALSE, "WRITE"=FALSE}, {"FUNCTION"="BCM_STAT_CENTRAL_LOCK\nCAN DATA", "READ"=FALSE, "WRITE"=FALSE}, {"FUNCTION"="BCM_STAT_DOOR_FLAP\nCAN DATA", "READ"=FALSE, "WRITE"=FALSE}, {"FUNCTION"="BCM_SunroofSts\nCAN DATA", "READ"=FALSE, "WRITE"=FALSE}, {"FUNCTION"="BCM_SunshadeSts\nCAN DATA", "READ"=FALSE, "WRITE"=FALSE}, {"FUNCTION"="BCM_SwitchSts\nCAN DATA", "READ"=FALSE, "WRITE"=FALSE}, {"FUNCTION"="BCM_TERMINAL\nCAN DATA", "READ"=FALSE, "WRITE"=FALSE}, {"FUNCTION"="BCM_VEHICLE_IDENT_NUMBER\nCAN DATA", "READ"=FALSE, "WRITE"=FALSE}, {"FUNCTION"="BCM_VOLTAGE\nCAN DATA", "READ"=FALSE, "WRITE"=FALSE}, {"FUNCTION"="BCM_WarnMsg\nCAN DATA", "READ"=FALSE, "WRITE"=FALSE}, {"FUNCTION"="BMS_CellTemp\nCAN DATA", "READ"=FALSE, "WRITE"=FALSE}, {"FUNCTION"="BMS_ChgParamReq\nCAN DATA", "READ"=FALSE, "WRITE"=FALSE}, {"FUNCTION"="BMS_CurMeas\nCAN DATA", "READ"=FALSE, "WRITE"=FALSE}, {"FUNCTION"="BMS_DiagReq\nCAN DATA", "READ"=FALSE, "WRITE"=FALSE}, {"FUNCTION"="BMS_DiagResp\nCAN DATA", "READ"=FALSE, "WRITE"=FALSE}, {"FUNCTION"="BMS_HVMeas1\nCAN DATA", "READ"=FALSE, "WRITE"=FALSE}, {"FUNCTION"="BMS_Sts\nCAN DATA", "READ"=FALSE, "WRITE"=FALSE}, {"FUNCTION"="BMS_WarnMsg\nCAN DATA", "READ"=FALSE, "WRITE"=FALSE}, {"FUNCTION"="CCUF_DiagReq\nCAN DATA", "READ"=FALSE, "WRITE"=FALSE}, {"FUNCTION"="CCUF_DiagResp\nCAN DATA", "READ"=FALSE, "WRITE"=FALSE}, {"FUNCTION"="CCUR_DiagReq\nCAN DATA", "READ"=FALSE, "WRITE"=FALSE}, {"FUNCTION"="CCUR_DiagResp\nCAN DATA", "READ"=FALSE, "WRITE"=FALSE}, {"FUNCTION"="CCU_STATUS\nCAN DATA", "READ"=FALSE, "WRITE"=FALSE}, {"FUNCTION"="CCU_TEMP_PRESSURE\nCAN DATA", "READ"=FALSE, "WRITE"=FALSE}, {"FUNCTION"="CCU_WarnMsg\nCAN DATA", "READ"=FALSE, "WRITE"=FALSE}, {"FUNCTION"="CPD_DiagReq\nCAN DATA", "READ"=FALSE, "WRITE"=FALSE}, {"FUNCTION"="CPD_DiagResp\nCAN DATA", "READ"=FALSE, "WRITE"=FALSE}, {"FUNCTION"="CPD_NM\nCAN DATA", "READ"=FALSE, "WRITE"=FALSE}, {"FUNCTION"="CPD_OUTPUT\nCAN DATA", "READ"=FALSE, "WRITE"=FALSE}, {"FUNCTION"="CPD_WarnMsg\nCAN DATA", "READ"=FALSE, "WRITE"=FALSE}, {"FUNCTION"="CPD_rDiagReq\nCAN DATA", "READ"=FALSE, "WRITE"=FALSE}, {"FUNCTION"="CPD_rDiagResp\nCAN DATA", "READ"=FALSE, "WRITE"=FALSE}, {"FUNCTION"="Camera_Lane\nCAN DATA", "READ"=FALSE, "WRITE"=FALSE}, {"FUNCTION"="Camera_Object01\nCAN DATA", "READ"=FALSE, "WRITE"=FALSE}, {"FUNCTION"="Camera_Object02\nCAN DATA", "READ"=FALSE, "WRITE"=FALSE}, {"FUNCTION"="Camera_Object03\nCAN DATA", "READ"=FALSE, "WRITE"=FALSE}, {"FUNCTION"="Camera_Object04\nCAN DATA", "READ"=FALSE, "WRITE"=FALSE}, {"FUNCTION"="Camera_Object05\nCAN DATA", "READ"=FALSE, "WRITE"=FALSE}, {"FUNCTION"="Camera_Object06\nCAN DATA", "READ"=FALSE, "WRITE"=FALSE}, {"FUNCTION"="Camera_leftlane\nCAN DATA", "READ"=FALSE, "WRITE"=FALSE}, {"FUNCTION"="Camera_rightlane\nCAN DATA", "READ"=FALSE, "WRITE"=FALSE}, {"FUNCTION"="DCM_APM_DiagReq\nCAN DATA", "READ"=FALSE, "WRITE"=FALSE}, {"FUNCTION"="DCM_APM_DiagResp\nCAN DATA", "READ"=FALSE, "WRITE"=FALSE}, {"FUNCTION"="DIAG_Req_All_CAN\nCAN DATA", "READ"=FALSE, "WRITE"=FALSE}, {"FUNCTION"="DIAG_Req_All_Ecu\nCAN DATA", "READ"=FALSE, "WRITE"=FALSE}, {"FUNCTION"="DIAG_Req_Info\nCAN DATA", "READ"=FALSE, "WRITE"=FALSE}, {"FUNCTION"="DMS_Status\nCAN DATA", "READ"=FALSE, "WRITE"=FALSE}, {"FUNCTION"="Diag_Request_ECU\nCAN DATA", "READ"=FALSE, "WRITE"=FALSE}, {"FUNCTION"="EASC_Confirm_sts\nCAN DATA", "READ"=FALSE, "WRITE"=FALSE}, {"FUNCTION"="EASC_DiagReq\nCAN DATA", "READ"=FALSE, "WRITE"=FALSE}, {"FUNCTION"="EASC_DiagResp\nCAN DATA", "READ"=FALSE, "WRITE"=FALSE}, {"FUNCTION"="EASC_NM\nCAN DATA", "READ"=FALSE, "WRITE"=FALSE}, {"FUNCTION"="EASC_WarnMsg\nCAN DATA", "READ"=FALSE, "WRITE"=FALSE}, {"FUNCTION"="EASC_rDiagReq\nCAN DATA", "READ"=FALSE, "WRITE"=FALSE}, {"FUNCTION"="EASC_rDiagResp\nCAN DATA", "READ"=FALSE, "WRITE"=FALSE}, {"FUNCTION"="EDS_F_DiagReq\nCAN DATA", "READ"=FALSE, "WRITE"=FALSE}, {"FUNCTION"="EDS_F_DiagResp\nCAN DATA", "READ"=FALSE, "WRITE"=FALSE}, {"FUNCTION"="EDS_F_WarnMsg\nCAN DATA", "READ"=FALSE, "WRITE"=FALSE}, {"FUNCTION"="EDS_OutPut_FR\nCAN DATA", "READ"=FALSE, "WRITE"=FALSE}, {"FUNCTION"="EDS_OutPut_RR\nCAN DATA", "READ"=FALSE, "WRITE"=FALSE}, {"FUNCTION"="EDS_R_DiagReq\nCAN DATA", "READ"=FALSE, "WRITE"=FALSE}, {"FUNCTION"="EDS_R_DiagResp\nCAN DATA", "READ"=FALSE, "WRITE"=FALSE}, {"FUNCTION"="EDS_R_WarnMsg\nCAN DATA", "READ"=FALSE, "WRITE"=FALSE}, {"FUNCTION"="EPS2_DiagReq\nCAN DATA", "READ"=FALSE, "WRITE"=FALSE}, {"FUNCTION"="EPS2_DiagResp\nCAN DATA", "READ"=FALSE, "WRITE"=FALSE}, {"FUNCTION"="EPS_DiagReq\nCAN DATA", "READ"=FALSE, "WRITE"=FALSE}, {"FUNCTION"="EPS_DiagResp\nCAN DATA", "READ"=FALSE, "WRITE"=FALSE}, {"FUNCTION"="EPS_WarnMsg\nCAN DATA", "READ"=FALSE, "WRITE"=FALSE}, {"FUNCTION"="ETG_DiagReq\nCAN DATA", "READ"=FALSE, "WRITE"=FALSE}, {"FUNCTION"="ETG_DiagResp\nCAN DATA", "READ"=FALSE, "WRITE"=FALSE}, {"FUNCTION"="ETG_STATUS\nCAN DATA", "READ"=FALSE, "WRITE"=FALSE}, {"FUNCTION"="ETG_WarnMsg\nCAN DATA", "READ"=FALSE, "WRITE"=FALSE}, {"FUNCTION"="GS_DiagReq\nCAN DATA", "READ"=FALSE, "WRITE"=FALSE}, {"FUNCTION"="GS_DiagResp\nCAN DATA", "READ"=FALSE, "WRITE"=FALSE}, {"FUNCTION"="GS_WarnMsg\nCAN DATA", "READ"=FALSE, "WRITE"=FALSE}, {"FUNCTION"="GW_BCM_Immo_MHU_Byte\nCAN DATA", "READ"=FALSE, "WRITE"=FALSE}, {"FUNCTION"="GW_BCM_RemoteCtrlSts\nCAN DATA", "READ"=FALSE, "WRITE"=FALSE}, {"FUNCTION"="HOD_Heating\nCAN DATA", "READ"=FALSE, "WRITE"=FALSE}, {"FUNCTION"="HOD_Heating_FDBK\nCAN DATA", "READ"=FALSE, "WRITE"=FALSE}, {"FUNCTION"="HUD_DiagReq\nCAN DATA", "READ"=FALSE, "WRITE"=FALSE}, {"FUNCTION"="HUD_DiagResp\nCAN DATA", "READ"=FALSE, "WRITE"=FALSE}, {"FUNCTION"="HUD_ECU_Status\nCAN DATA", "READ"=FALSE, "WRITE"=FALSE}, {"FUNCTION"="HUD_NM\nCAN DATA", "READ"=FALSE, "WRITE"=FALSE}, {"FUNCTION"="HUD_State\nCAN DATA", "READ"=FALSE, "WRITE"=FALSE}, {"FUNCTION"="HUD_WarnMsg\nCAN DATA", "READ"=FALSE, "WRITE"=FALSE}, {"FUNCTION"="HUD_rDiagReq\nCAN DATA", "READ"=FALSE, "WRITE"=FALSE}, {"FUNCTION"="HUD_rDiagResp\nCAN DATA", "READ"=FALSE, "WRITE"=FALSE}, {"FUNCTION"="IC_BORD_COMP_TRIP_A\nCAN DATA", "READ"=FALSE, "WRITE"=FALSE}, {"FUNCTION"="IC_BORD_COMP_TRIP_Auto\nCAN DATA", "READ"=FALSE, "WRITE"=FALSE}, {"FUNCTION"="IC_BORD_COMP_TRIP_B\nCAN DATA", "READ"=FALSE, "WRITE"=FALSE}, {"FUNCTION"="IC_MILEAGE\nCAN DATA", "READ"=FALSE, "WRITE"=FALSE}, {"FUNCTION"="IC_ODO\nCAN DATA", "READ"=FALSE, "WRITE"=FALSE}, {"FUNCTION"="IC_RELATIVIME\nCAN DATA", "READ"=FALSE, "WRITE"=FALSE}, {"FUNCTION"="IC_SENSOR\nCAN DATA", "READ"=FALSE, "WRITE"=FALSE}, {"FUNCTION"="IC_STAT_AIRBAG\nCAN DATA", "READ"=FALSE, "WRITE"=FALSE}, {"FUNCTION"="IDB_ACC_LONG_LAT_YAW\nCAN DATA", "READ"=FALSE, "WRITE"=FALSE}, {"FUNCTION"="IDB_DiagReq\nCAN DATA", "READ"=FALSE, "WRITE"=FALSE}, {"FUNCTION"="IDB_DiagResp\nCAN DATA", "READ"=FALSE, "WRITE"=FALSE}, {"FUNCTION"="IDB_EPB_STATUS\nCAN DATA", "READ"=FALSE, "WRITE"=FALSE}, {"FUNCTION"="IDB_FUNCTION\nCAN DATA", "READ"=FALSE, "WRITE"=FALSE}, {"FUNCTION"="IDB_MILEAGE\nCAN DATA", "READ"=FALSE, "WRITE"=FALSE}, {"FUNCTION"="IDB_STATUS\nCAN DATA", "READ"=FALSE, "WRITE"=FALSE}, {"FUNCTION"="IDB_V_VEH\nCAN DATA", "READ"=FALSE, "WRITE"=FALSE}, {"FUNCTION"="IDB_WarnMsg\nCAN DATA", "READ"=FALSE, "WRITE"=FALSE}, {"FUNCTION"="LDML_LIGHT\nCAN DATA", "READ"=FALSE, "WRITE"=FALSE}, {"FUNCTION"="LDMR_LIGHT\nCAN DATA", "READ"=FALSE, "WRITE"=FALSE}, {"FUNCTION"="LDM_L_DiagReq\nCAN DATA", "READ"=FALSE, "WRITE"=FALSE}, {"FUNCTION"="LDM_L_DiagResp\nCAN DATA", "READ"=FALSE, "WRITE"=FALSE}, {"FUNCTION"="LDM_R_DiagReq\nCAN DATA", "READ"=FALSE, "WRITE"=FALSE}, {"FUNCTION"="LDM_R_DiagResp\nCAN DATA", "READ"=FALSE, "WRITE"=FALSE}, {"FUNCTION"="MFS_Control_Button\nCAN DATA", "READ"=FALSE, "WRITE"=FALSE}, {"FUNCTION"="MHU_ADAS_RP_Ctrl\nCAN DATA", "READ"=FALSE, "WRITE"=FALSE}, {"FUNCTION"="MHU_ADAS_RSSI\nCAN DATA", "READ"=FALSE, "WRITE"=FALSE}, {"FUNCTION"="MHU_ADAS_req\nCAN DATA", "READ"=FALSE, "WRITE"=FALSE}, {"FUNCTION"="MHU_AMP_Ann1_ModeSET\nCAN DATA", "READ"=FALSE, "WRITE"=FALSE}, {"FUNCTION"="MHU_AMP_Ann1_PromptsSET\nCAN DATA", "READ"=FALSE, "WRITE"=FALSE}, {"FUNCTION"="MHU_AMP_Ann2_SpeakerSET\nCAN DATA", "READ"=FALSE, "WRITE"=FALSE}, {"FUNCTION"="MHU_AmpEQType\nCAN DATA", "READ"=FALSE, "WRITE"=FALSE}, {"FUNCTION"="MHU_AmpSET\nCAN DATA", "READ"=FALSE, "WRITE"=FALSE}, {"FUNCTION"="MHU_Auth_Immo\nCAN DATA", "READ"=FALSE, "WRITE"=FALSE}, {"FUNCTION"="MHU_Auth_Immo_ADAS\nCAN DATA", "READ"=FALSE, "WRITE"=FALSE}, {"FUNCTION"="MHU_Avas_Setting\nCAN DATA", "READ"=FALSE, "WRITE"=FALSE}, {"FUNCTION"="MHU_BCM_Color_Req\nCAN DATA", "READ"=FALSE, "WRITE"=FALSE}, {"FUNCTION"="MHU_BCM_DoorsCtrl\nCAN DATA", "READ"=FALSE, "WRITE"=FALSE}, {"FUNCTION"="MHU_BCM_HornLightControl\nCAN DATA", "READ"=FALSE, "WRITE"=FALSE}, {"FUNCTION"="MHU_BCM_IntensityTiming_Req\nCAN DATA", "READ"=FALSE, "WRITE"=FALSE}, {"FUNCTION"="MHU_BCM_RemoteClampCtrl\nCAN DATA", "READ"=FALSE, "WRITE"=FALSE}, {"FUNCTION"="MHU_CCUF_ClimateSetting\nCAN DATA", "READ"=FALSE, "WRITE"=FALSE}, {"FUNCTION"="MHU_CCUR_ClimateSetting\nCAN DATA", "READ"=FALSE, "WRITE"=FALSE}, {"FUNCTION"="MHU_CPD_Confirm\nCAN DATA", "READ"=FALSE, "WRITE"=FALSE}, {"FUNCTION"="MHU_CarMode_Switch\nCAN DATA", "READ"=FALSE, "WRITE"=FALSE}, {"FUNCTION"="MHU_ComfortSetting\nCAN DATA", "READ"=FALSE, "WRITE"=FALSE}, {"FUNCTION"="MHU_DATE_TIME\nCAN DATA", "READ"=FALSE, "WRITE"=FALSE}, {"FUNCTION"="MHU_DIGIT_SPEED\nCAN DATA", "READ"=FALSE, "WRITE"=FALSE}, {"FUNCTION"="MHU_DMS_STATUS\nCAN DATA", "READ"=FALSE, "WRITE"=FALSE}, {"FUNCTION"="MHU_DRIVER_INFO\nCAN DATA", "READ"=FALSE, "WRITE"=FALSE}, {"FUNCTION"="MHU_DiagReq\nCAN DATA", "READ"=FALSE, "WRITE"=FALSE}, {"FUNCTION"="MHU_DiagResp\nCAN DATA", "READ"=FALSE, "WRITE"=FALSE}, {"FUNCTION"="MHU_DoorSetting\nCAN DATA", "READ"=FALSE, "WRITE"=FALSE}, {"FUNCTION"="MHU_EvSetting\nCAN DATA", "READ"=FALSE, "WRITE"=FALSE}, {"FUNCTION"="MHU_FEEDBACK_APA\nCAN DATA", "READ"=FALSE, "WRITE"=FALSE}, {"FUNCTION"="MHU_FOTA_ReqAll\nCAN DATA", "READ"=FALSE, "WRITE"=FALSE}, {"FUNCTION"="MHU_FOTA_STATUS\nCAN DATA", "READ"=FALSE, "WRITE"=FALSE}, {"FUNCTION"="MHU_HEADLAMP_CTL\nCAN DATA", "READ"=FALSE, "WRITE"=FALSE}, {"FUNCTION"="MHU_HUD_BASE\nCAN DATA", "READ"=FALSE, "WRITE"=FALSE}, {"FUNCTION"="MHU_HUD_Info_1\nCAN DATA", "READ"=FALSE, "WRITE"=FALSE}, {"FUNCTION"="MHU_HUD_NAV_DISP\nCAN DATA", "READ"=FALSE, "WRITE"=FALSE}, {"FUNCTION"="MHU_HUD_NAV_GuidanceCont\nCAN DATA", "READ"=FALSE, "WRITE"=FALSE}, {"FUNCTION"="MHU_HudPositionSetting\nCAN DATA", "READ"=FALSE, "WRITE"=FALSE}, {"FUNCTION"="MHU_HudSetting\nCAN DATA", "READ"=FALSE, "WRITE"=FALSE}, {"FUNCTION"="MHU_IDB_Mode_Select\nCAN DATA", "READ"=FALSE, "WRITE"=FALSE}, {"FUNCTION"="MHU_ISA_Speed\nCAN DATA", "READ"=FALSE, "WRITE"=FALSE}, {"FUNCTION"="MHU_LightSetting\nCAN DATA", "READ"=FALSE, "WRITE"=FALSE}, {"FUNCTION"="MHU_MirrorAdjust\nCAN DATA", "READ"=FALSE, "WRITE"=FALSE}, {"FUNCTION"="MHU_NAV_JUNC_INFO\nCAN DATA", "READ"=FALSE, "WRITE"=FALSE}, {"FUNCTION"="MHU_NM\nCAN DATA", "READ"=FALSE, "WRITE"=FALSE}, {"FUNCTION"="MHU_SEAT_CONTROL\nCAN DATA", "READ"=FALSE, "WRITE"=FALSE}, {"FUNCTION"="MHU_STATUS\nCAN DATA", "READ"=FALSE, "WRITE"=FALSE}, {"FUNCTION"="MHU_SeatVentHeat\nCAN DATA", "READ"=FALSE, "WRITE"=FALSE}, {"FUNCTION"="MHU_SteeringAdjust\nCAN DATA", "READ"=FALSE, "WRITE"=FALSE}, {"FUNCTION"="MHU_UserProfile\nCAN DATA", "READ"=FALSE, "WRITE"=FALSE}, {"FUNCTION"="MHU_WindowSetting\nCAN DATA", "READ"=FALSE, "WRITE"=FALSE}, {"FUNCTION"="MRGEN_DiagReq\nCAN DATA", "READ"=FALSE, "WRITE"=FALSE}, {"FUNCTION"="MRGEN_DiagResp\nCAN DATA", "READ"=FALSE, "WRITE"=FALSE}, {"FUNCTION"="OCS_P_DiagReq\nCAN DATA", "READ"=FALSE, "WRITE"=FALSE}, {"FUNCTION"="OCS_P_DiagResp\nCAN DATA", "READ"=FALSE, "WRITE"=FALSE}, {"FUNCTION"="POD_DCDC_DiagReq\nCAN DATA", "READ"=FALSE, "WRITE"=FALSE}, {"FUNCTION"="POD_DCDC_DiagResp\nCAN DATA", "READ"=FALSE, "WRITE"=FALSE}, {"FUNCTION"="POD_GW_Request\nCAN DATA", "READ"=FALSE, "WRITE"=FALSE}, {"FUNCTION"="POD_GW_Response\nCAN DATA", "READ"=FALSE, "WRITE"=FALSE}, {"FUNCTION"="POD_OBC_DiagReq\nCAN DATA", "READ"=FALSE, "WRITE"=FALSE}, {"FUNCTION"="POD_OBC_DiagResp\nCAN DATA", "READ"=FALSE, "WRITE"=FALSE}, {"FUNCTION"="POD_WarnMsg\nCAN DATA", "READ"=FALSE, "WRITE"=FALSE}, {"FUNCTION"="PSM_D_DiagReq\nCAN DATA", "READ"=FALSE, "WRITE"=FALSE}, {"FUNCTION"="PSM_D_DiagResp\nCAN DATA", "READ"=FALSE, "WRITE"=FALSE}, {"FUNCTION"="PSM_D_SEAT_CONTROL\nCAN DATA", "READ"=FALSE, "WRITE"=FALSE}, {"FUNCTION"="PSM_SEAT_POSITION\nCAN DATA", "READ"=FALSE, "WRITE"=FALSE}, {"FUNCTION"="PSM_WarnMsg\nCAN DATA", "READ"=FALSE, "WRITE"=FALSE}, {"FUNCTION"="RCU_DiagReq\nCAN DATA", "READ"=FALSE, "WRITE"=FALSE}, {"FUNCTION"="RCU_DiagResp\nCAN DATA", "READ"=FALSE, "WRITE"=FALSE}, {"FUNCTION"="RCU_WarnMsg\nCAN DATA", "READ"=FALSE, "WRITE"=FALSE}, {"FUNCTION"="SAS_Sensor\nCAN DATA", "READ"=FALSE, "WRITE"=FALSE}, {"FUNCTION"="SCAM_DiagReq\nCAN DATA", "READ"=FALSE, "WRITE"=FALSE}, {"FUNCTION"="SCAM_DiagResp\nCAN DATA", "READ"=FALSE, "WRITE"=FALSE}, {"FUNCTION"="SCM_Raw_Status\nCAN DATA", "READ"=FALSE, "WRITE"=FALSE}, {"FUNCTION"="SHVU_F_Confirm_Sts\nCAN DATA", "READ"=FALSE, "WRITE"=FALSE}, {"FUNCTION"="SHVU_F_DiagReq\nCAN DATA", "READ"=FALSE, "WRITE"=FALSE}, {"FUNCTION"="SHVU_F_DiagResp\nCAN DATA", "READ"=FALSE, "WRITE"=FALSE}, {"FUNCTION"="SHVU_R_Confirm_Sts\nCAN DATA", "READ"=FALSE, "WRITE"=FALSE}, {"FUNCTION"="SHVU_R_DiagReq\nCAN DATA", "READ"=FALSE, "WRITE"=FALSE}, {"FUNCTION"="SHVU_R_DiagResp\nCAN DATA", "READ"=FALSE, "WRITE"=FALSE}, {"FUNCTION"="SRR_FL_DiagReq\nCAN DATA", "READ"=FALSE, "WRITE"=FALSE}, {"FUNCTION"="SRR_FL_DiagResp\nCAN DATA", "READ"=FALSE, "WRITE"=FALSE}, {"FUNCTION"="SRR_FR_DiagReq\nCAN DATA", "READ"=FALSE, "WRITE"=FALSE}, {"FUNCTION"="SRR_FR_DiagResp\nCAN DATA", "READ"=FALSE, "WRITE"=FALSE}, {"FUNCTION"="SRR_RL_DiagReq\nCAN DATA", "READ"=FALSE, "WRITE"=FALSE}, {"FUNCTION"="SRR_RL_DiagResp\nCAN DATA", "READ"=FALSE, "WRITE"=FALSE}, {"FUNCTION"="SRR_RR_DiagReq\nCAN DATA", "READ"=FALSE, "WRITE"=FALSE}, {"FUNCTION"="SRR_RR_DiagResp\nCAN DATA", "READ"=FALSE, "WRITE"=FALSE}, {"FUNCTION"="SeatMassage_Input\nCAN DATA", "READ"=FALSE, "WRITE"=FALSE}, {"FUNCTION"="SeatMassage_Output\nCAN DATA", "READ"=FALSE, "WRITE"=FALSE}, {"FUNCTION"="Sensor_Fault\nCAN DATA", "READ"=FALSE, "WRITE"=FALSE}, {"FUNCTION"="TPMS_TirePressure\nCAN DATA", "READ"=FALSE, "WRITE"=FALSE}, {"FUNCTION"="TRM_DiagReq\nCAN DATA", "READ"=FALSE, "WRITE"=FALSE}, {"FUNCTION"="TRM_DiagResp\nCAN DATA", "READ"=FALSE, "WRITE"=FALSE}, {"FUNCTION"="TRM_WarnMsg\nCAN DATA", "READ"=FALSE, "WRITE"=FALSE}, {"FUNCTION"="VCU_ChargingConnection\nCAN DATA", "READ"=FALSE, "WRITE"=FALSE}, {"FUNCTION"="VCU_DiagReq\nCAN DATA", "READ"=FALSE, "WRITE"=FALSE}, {"FUNCTION"="VCU_DiagResp\nCAN DATA", "READ"=FALSE, "WRITE"=FALSE}, {"FUNCTION"="VCU_HMI_Info\nCAN DATA", "READ"=FALSE, "WRITE"=FALSE}, {"FUNCTION"="VCU_HV_DrvSys_status\nCAN DATA", "READ"=FALSE, "WRITE"=FALSE}, {"FUNCTION"="VCU_HVsystem_status\nCAN DATA", "READ"=FALSE, "WRITE"=FALSE}, {"FUNCTION"="VCU_MHU_info\nCAN DATA", "READ"=FALSE, "WRITE"=FALSE}, {"FUNCTION"="VCU_WarnMsg\nCAN DATA", "READ"=FALSE, "WRITE"=FALSE}, {"FUNCTION"="WLC_Status\nCAN DATA", "READ"=FALSE, "WRITE"=FALSE}, {"FUNCTION"="WLC_Status_2\nCAN DATA", "READ"=FALSE, "WRITE"=FALSE}, {"FUNCTION"="XGW_DiagReq\nCAN DATA", "READ"=FALSE, "WRITE"=FALSE}, {"FUNCTION"="XGW_DiagResp\nCAN DATA", "READ"=FALSE, "WRITE"=FALSE}, {"FUNCTION"="XGW_FOTA_StsConfirm\nCAN DATA", "READ"=FALSE, "WRITE"=FALSE}, {"FUNCTION"="XGW_HCMInfo\nCAN DATA", "READ"=FALSE, "WRITE"=FALSE}, {"FUNCTION"="XGW_Info_Collect\nCAN DATA", "READ"=FALSE, "WRITE"=FALSE}, {"FUNCTION"="XGW_NM\nCAN DATA", "READ"=FALSE, "WRITE"=FALSE}, {"FUNCTION"="XGW_System_Info\nCAN DATA", "READ"=FALSE, "WRITE"=FALSE}, {"FUNCTION"="XGW_WarnMsg\nCAN DATA", "READ"=FALSE, "WRITE"=FALSE}, {"FUNCTION"="YSS_DiagReq\nCAN DATA", "READ"=FALSE, "WRITE"=FALSE}, {"FUNCTION"="YSS_DiagResp\nCAN DATA", "READ"=FALSE, "WRITE"=FALSE}]  # ALL DBC FUNCTIONS
        w155 = T8 {"Current VI Reference"=refnum, "Close Panel on Exit?"=FALSE}  # Core
        w157 = TRUE  # Your Boolean data
        w156 = ""  # Your string data
        # "do not delete - used by framework"
        # "Data names and types of shift register data are defined by this bundle."
        # "Initialize the shift-register data, here.\n(data names are defined by what you wire into the bundle function)"
        n67 = Bundle("Core"=w155, "Your Boolean data"=w157, "Your string data"=w156, "ALL DBC FUNCTIONS"=w154, "File paths"=w153, "DBC FUNCTIONS"=w152) -> (w159:T6)  [unwired: 1 in]
        n68 = call <vilib>:"Add State(s) to Queue__JKI_lib_State_Machine.vi"("State(s) in (\"\")"=w161) -> ("States Out"=w160:string)  [unwired: 14 in]
      }
      frame "Data: Cleanup" {
        # "Cleanup any data and references, here.\n(this is called automatically, by the Macro: Exit)"
        n69 = Unbundle By Name(w162) -> ("Core.Current VI Reference"=w165:refnum<vi>)
        n70 = Close Reference(reference=w165, error in (no error)=w164) -> (error out=w163:errorcluster)
        n71 = call <vilib>:"Add State(s) to Queue__JKI_lib_State_Machine.vi"("State(s) in (\"\")"=w167) -> ("States Out"=w166:string)  [unwired: 14 in]
      }
      frame "---------- Events ----------" {
        # "Do not put any code in this frame.\n(It is a separator no-op. You can make a copy of this frame to create a new UI frame)"
        n72 = call <vilib>:"Add State(s) to Queue__JKI_lib_State_Machine.vi"("State(s) in (\"\")"=w171) -> ("States Out"=w170:string)  [unwired: 14 in]
      }
      frame "Events: Register" {
        # "Do not put any code in this frame.\n(It is a separator no-op. You can make a copy of this frame to create a new UI frame)"
        n73 = call <vilib>:"Add State(s) to Queue__JKI_lib_State_Machine.vi"("State(s) in (\"\")"=w175) -> ("States Out"=w174:string)  [unwired: 14 in]
      }
      frame "Events: Unregister" {
        # "Do not put any code in this frame.\n(It is a separator no-op. You can make a copy of this frame to create a new UI frame)"
        n74 = Unregister For Events(event registration refnum=w178, error in=w177) -> (error out=w176:errorcluster)
        n75 = call <vilib>:"Add State(s) to Queue__JKI_lib_State_Machine.vi"("State(s) in (\"\")"=w181) -> ("States Out"=w180:string)  [unwired: 14 in]
      }
      frame "---------- UI ----------" {
        # "Do not put any code in this frame.\n(It is a separator no-op. You can make a copy of this frame to create a new UI frame)"
        n76 = call <vilib>:"Add State(s) to Queue__JKI_lib_State_Machine.vi"("State(s) in (\"\")"=w185) -> ("States Out"=w184:string)  [unwired: 14 in]
      }
      frame "UI: Initialize" {
        # "Initialize the User Interface, here.\n(this is called automatically, by the Macro: Init)"
        n77 = invoke class="VI" method="Default Vals.Reinit All"(error in=w190) -> (error out=w189:errorcluster)  [unwired: 2 in, 2 out]
        n78 = Current VI's Path() -> (path=w195:path)
        n79 = call "FEV_Strip & Build Path.vi"("Strip Levels"=2, "error in (no error)"=w189, "Build Path"="Data\\Models", "Path In"=w195) -> ("error out"=w193:errorcluster, "New Path Out"=w187:path)  [unwired: 5 in, 1 out]
        n80 = List Folder(path=w187) -> (folder names=w186:string[])  [unwired: 3 in, 3 out]
        n81 = Bundle By Name(cluster=w192, "File paths.Base file path"=w187) -> (w191:T6)
        n82 = property on="MODEL SELECTION" class="CmbBox"("Strings[]"=w186) -> ()  [unwired: 2 in, 2 out]
        n83 = call <vilib>:"Add State(s) to Queue__JKI_lib_State_Machine.vi"("State(s) in (\"\")"=w198) -> ("States Out"=w197:string)  [unwired: 14 in]
        "Headline" <- "CAN Configuration" ("Headline")
      }
      frame "UI: Cursor Set" {
        # "Argument"
        # "Set and Unset Cursor Busy.\n(Usage: \"UI: Cursor Set >> Busy|Idle\")"
        n84 = case shown="\"Idle\", Default" w199 {
          tunnel: w201 -> [w206 w208]
          tunnel: [w205 w207] -> w200
          frame "Idle", Default {
            n85 = call <vilib>:"Unset Busy.vi"("error in (no error)"=w206) -> ("error out"=w205:errorcluster)  [unwired: 10 in]
          }
          frame "Busy" {
            n86 = call <vilib>:"Set Busy.vi"("error in (no error)"=w208) -> ("error out"=w207:errorcluster)  [unwired: 9 in, 1 out]
          }
        }
        n87 = call <vilib>:"Add State(s) to Queue__JKI_lib_State_Machine.vi"("State(s) in (\"\")"=w204) -> ("States Out"=w203:string)  [unwired: 14 in]
      }
      frame "UI: Front Panel State" {
        # "Argument"
        # "Set Front Panel Open or Closed\n(Usage: \"UI: Front Panel State >> Open|Close\")"
        n88 = Unbundle By Name(w211) -> ("Core.Current VI Reference"=w210:refnum<vi>)
        n89 = case shown="\"Open\", \"Standard\", Default" w209 {
          tunnel: w213 -> [w221 w236 w247 w260 w273]
          tunnel: [w223 w237 w249 w262 w275] -> w212
          tunnel: w210 -> [w222 w234 w248 w261 w274]
          frame "Open", "Standard", Default {
            w216 = T4."Standard" ("State")
            n90 = property class="VI"(reference=w222, error in=w221) -> (reference out=w219:refnum<vi>, error out=w220:errorcluster, "FP.State"=w218:T4)
            n91 = Not Equal?(x=w218, y=w216) -> (x != y?=w217:bool)
            n92 = case shown="True" w217 {
              tunnel: [w227 w229] -> w223
              tunnel: w220 -> [w226 w229]
              tunnel: w219 -> [w225 _]
              tunnel: w216 -> [w224 _]
              frame True {
                n93 = invoke class="VI" method="FP.Open"(reference=w225, error in=w226, "Activate"=TRUE, "State"=w224) -> (error out=w227:errorcluster)  [unwired: 1 in, 4 out]
              }
              frame False {
              }
            }
          }
          frame "Close", "Closed" {
            n94 = property class="VI"(reference=w234, error in=w236) -> (reference out=w233:refnum<vi>, error out=w235:errorcluster, "FP.State"=w231:T4)
            n95 = Not Equal?(x=w231, y=T4."Closed" ("Front Panel Window:State")) -> (x != y?=w230:bool)
            n96 = case shown="True" w230 {
              tunnel: [w238 w241] -> w237
              tunnel: w235 -> [w238 w240]
              tunnel: w233 -> [_ w239]
              frame False {
              }
              frame True {
                n97 = invoke class="VI" method="FP.Close"(reference=w239, error in=w240) -> (error out=w241:errorcluster)  [unwired: 1 in, 2 out]
              }
            }
          }
          frame "Hidden", "Hide" {
            w242 = T4."Hidden" ("State")
            n98 = property class="VI"(reference=w248, error in=w247) -> (reference out=w245:refnum<vi>, error out=w246:errorcluster, "FP.State"=w244:T4)
            n99 = Not Equal?(x=w244, y=w242) -> (x != y?=w243:bool)
            n100 = case shown="True" w243 {
              tunnel: [w253 w254] -> w249
              tunnel: w246 -> [w252 w254]
              tunnel: w245 -> [w251 _]
              tunnel: w242 -> [w250 _]
              frame True {
                n101 = invoke class="VI" method="FP.Open"(reference=w251, error in=w252, "State"=w250) -> (error out=w253:errorcluster)  [unwired: 2 in, 4 out]
              }
              frame False {
              }
            }
          }
          frame "Minimize", "Minimized" {
            w255 = T4."Minimized" ("State")
            n102 = property class="VI"(reference=w261, error in=w260) -> (reference out=w258:refnum<vi>, error out=w259:errorcluster, "FP.State"=w257:T4)
            n103 = Not Equal?(x=w257, y=w255) -> (x != y?=w256:bool)
            n104 = case shown="True" w256 {
              tunnel: [w266 w267] -> w262
              tunnel: w259 -> [w265 w267]
              tunnel: w258 -> [w264 _]
              tunnel: w255 -> [w263 _]
              frame True {
                n105 = invoke class="VI" method="FP.Open"(reference=w264, error in=w265, "State"=w263) -> (error out=w266:errorcluster)  [unwired: 2 in, 4 out]
              }
              frame False {
              }
            }
          }
          frame "Maximize", "Maximized" {
            w268 = T4."Maximized" ("State")
            n106 = property class="VI"(reference=w274, error in=w273) -> (reference out=w271:refnum<vi>, error out=w272:errorcluster, "FP.State"=w270:T4)
            n107 = Not Equal?(x=w270, y=w268) -> (x != y?=w269:bool)
            n108 = case shown="True" w269 {
              tunnel: [w279 w280] -> w275
              tunnel: w272 -> [w278 w280]
              tunnel: w271 -> [w277 _]
              tunnel: w268 -> [w276 _]
              frame True {
                n109 = invoke class="VI" method="FP.Open"(reference=w277, error in=w278, "State"=w276) -> (error out=w279:errorcluster)  [unwired: 2 in, 4 out]
              }
              frame False {
              }
            }
          }
        }
        n110 = call <vilib>:"Add State(s) to Queue__JKI_lib_State_Machine.vi"("State(s) in (\"\")"=w215) -> ("States Out"=w214:string)  [unwired: 14 in]
      }
      frame "---------- Macro ----------" {
        # "Do not put any code in this frame.\n(It is a separator no-op. You can make a copy of this frame to create a new Macro frame)"
        n111 = call <vilib>:"Add State(s) to Queue__JKI_lib_State_Machine.vi"("State(s) in (\"\")"=w284) -> ("States Out"=w283:string)  [unwired: 14 in]
      }
      frame "Macro: Initialize" {
        # "Initialization Macro\n(This is called once, when the VI starts)"
        n112 = call <vilib>:"Add State(s) to Queue__JKI_lib_State_Machine.vi"("State(s) in Front (\"\")"="Data: Initialize\nInitialize Core Data\nEvents: Register\nUI: Initialize\nUI: Front Panel State >> Open", "State(s) in (\"\")"=w289) -> ("States Out"=w288:string)  [unwired: 13 in]
      }
      frame "Macro: Exit" {
        # "Exit Macro\n(This is called once, when the VI exits)"
        n113 = Unbundle By Name(w296) -> ("Core.Close Panel on Exit?"=w295:bool)
        n114 = Select(t="UI: Front Panel State >> Close", s=w295, f="") -> (s? t:f=w292:string)
        n115 = call <vilib>:"Add State(s) to Queue__JKI_lib_State_Machine.vi"("State(s) in (\"\")"=w292, "State(s) at Back (\"\")"="Data: Cleanup\nEvents: Unregister\nExit") -> ("States Out"=w290:string)  [unwired: 13 in]
        n116 = call <vilib>:"Add State(s) to Queue__JKI_lib_State_Machine.vi"("State(s) in Front (\"\")"=w290, "State(s) in (\"\")"=w299) -> ("States Out"=w298:string)  [unwired: 13 in]
      }
      frame "---------- DATABSE ----------" {
        # "Template Separator\n(You can make a copy of, or modify, this frame)"
        n117 = call <vilib>:"Add State(s) to Queue__JKI_lib_State_Machine.vi"("State(s) in (\"\")"=w303) -> ("States Out"=w302:string)  [unwired: 14 in]
      }
      frame "DATABASE: SAVE DATABASE" {
        # "Your code here.\n(You can make a copy of, or modify, this frame)"
        n118 = Unbundle By Name(w315) -> ("DBC FUNCTIONS"=w307:T1[], "ALL DBC FUNCTIONS"=w304:T3[], "File paths.Model File path"=w310:path)
        n119 = Build Path(base path=w310, name or relative path="ALL DBC.txt") -> (appended path=w312:path)
        "appended path" <- w312
        n120 = Build Path(base path=w310, name or relative path="DBC FUNCTION.txt") -> (appended path=w308:path)
        n121 = Write to Binary File(file (use dialog)=w312, data=w304, error in=w314) -> (error out=w311:errorcluster)  [unwired: 3 in, 2 out]
        n122 = Write to Binary File(file (use dialog)=w308, data=w307, error in=w311) -> (error out=w305:errorcluster)  [unwired: 3 in, 2 out]
        n123 = flat-sequence {
          tunnel: [w319] -> w306
          tunnel: w305 -> [w319]
          frame #0 {
            n124 = One Button Dialog(message="DBC data is Saved") -> ()  [unwired: 1 in, 1 out]
          }
        }
        n125 = call <vilib>:"Add State(s) to Queue__JKI_lib_State_Machine.vi"("State(s) in (\"\")"=w317) -> ("States Out"=w316:string)  [unwired: 14 in]
      }
      frame "DATABASE: READ DATABASE" {
        # "Your code here.\n(You can make a copy of, or modify, this frame)"
        n126 = Unbundle By Name(w336) -> ("DBC FUNCTIONS"=w321:T1[], "ALL DBC FUNCTIONS"=w337:T3[], "File paths.Model File path"=w327:path)
        "File paths.Model File path" <- w327
        n127 = Build Path(base path=w327, name or relative path="DBC FUNCTION.txt") -> (appended path=w326:path)
        n128 = Build Path(base path=w327, name or relative path="ALL DBC.txt") -> (appended path=w332:path)
        n129 = call <vilib>:"Check if File or Folder Exists.vi"("error in (no error)"=w325, "path"=w326) -> ("error out"=w324:errorcluster, "file or folder exists?"=w322:bool, "dup path"=w323:path)  [unwired: 7 in]
        n130 = call <vilib>:"Check if File or Folder Exists.vi"("error in (no error)"=w325, "path"=w332) -> ("error out"=w330:errorcluster, "file or folder exists?"=w329:bool, "dup path"=w331:path)  [unwired: 7 in]
        n131 = case shown="True" w329 {
          tunnel: w337 -> [w350 w356]
          tunnel: [w349 w354] -> w334
          tunnel: [w350 w353] -> w333
          tunnel: w331 -> [_ w352]
          tunnel: w330 -> [w349 w351]
          frame False {
          }
          frame True {
            n132 = Read from Binary File(5:w356, 8:w351, 11:w352) -> (0:w355:errorcluster, 2:w353:T3[])  [unwired: 3 in, 2 out]
            n133 = property on="ALL DBC FUNCTIONS" class="Arr (strict)"(error in=w355, "Value"=w353) -> (error out=w354:errorcluster)  [unwired: 1 in, 1 out]
          }
        }
        n134 = case shown="True" w322 {
          tunnel: w321 -> [w342 w348]
          tunnel: [w341 w344] -> _
          tunnel: [w342 w343] -> w320
          tunnel: w323 -> [_ w347]
          tunnel: w324 -> [w341 w346]
          frame False {
          }
          frame True {
            n135 = Read from Binary File(5:w348, 8:w346, 11:w347) -> (0:w345:errorcluster, 2:w343:T1[])  [unwired: 3 in, 2 out]
            n136 = property on="DBC FUNCTIONS" class="Arr (strict)"(error in=w345, "Value"=w343) -> (error out=w344:errorcluster)  [unwired: 1 in, 1 out]
          }
        }
        n137 = Bundle By Name(cluster=w336, "ALL DBC FUNCTIONS"=w333, "DBC FUNCTIONS"=w320) -> (w335:T6)
        n138 = call <vilib>:"Add State(s) to Queue__JKI_lib_State_Machine.vi"("State(s) in (\"\")"=w340) -> ("States Out"=w339:string)  [unwired: 14 in]
      }
    }
  }
